vi "Buncher.vi"() -> ()   [LabVIEW 2014, in "Panels.lvlib"]
uses:
  Panels.lvlib
  CSlibraries-extern/DimLVEvent/DimIndicators/DimIndicators.lvlib
  CSlibraries/UtilityLib/UtilityLib.lvlib
  CS_Core/CSSystem/CoreLib/CoreLib.lvlib
  CSlibraries/UtilityLib/UtilityLib.valueStatus.ctl
  CS_Core/CSSystem/CoreLib/CoreLib.string 2 byte array.vi
  CSlibraries-extern/DimLVEvent/LVDimInterface/LVDimInterface.lvlib
  Instance           1 15Saved   Buncher .vi
  CS_Core/CSSystem/CoreLib/CoreLib.double 2 byte array.vi
  CS_Core/CSSystem/CoreLib/CoreLib.short 2 byte array.vi
  CSlibraries-extern/DimLVEvent/DimIndicators/DimIndicators.numericType.ctl
  CS_Core/BaseProcess/BaseProcess.descriptor string definition.ctl
  CS_Core/BaseProcess/BaseProcess.lvlib
  CS_Core/CSSystem/CoreDefs/CoreDefs.rawDataType.ctl
  CS_Core/CSSystem/CoreDefs/CoreDefs.call_type.ctl
  CSlibraries-extern/DimLVEvent/DimIndicators/DimIndicators.numericArrayType.ctl
  CSlibraries-extern/DimLVEvent/DimIndicators/DimIndicators.anyType.ctl
panel:
  in  "ListOfBases_Data":T1={"data"="NOLINK", "no link"=TRUE, "quality"=-1, "timeStamp"=0.0}
  in  "AmpCool":bool
  in  "AmpMicro":bool
  in  "AmpBun":bool
  in  "PercentNeon_SetValueInfoData":T2={"data"=[], "no link"=TRUE, "quality"=-1, "timeStamp"=0.0}
  in  "PercentNeon_SetData":T2={"data"=[], "no link"=TRUE, "quality"=-1, "timeStamp"=0.0}
  in  "PercentNeon":dbl=inf
  in  "SetFileLocation_Data":T1={"data"="NOLINK", "no link"=TRUE, "quality"=-1, "timeStamp"=0.0}
  in  "CoolPress":bool
  out "CoolPress_Mon":dbl=inf format="%.4f"
  in  "bunBase_SetValueInfoData":T2={"data"=[], "no link"=TRUE, "quality"=-1, "timeStamp"=0.0}
  in  "BunDefY_SetValueInfoData":T2={"data"=[], "no link"=TRUE, "quality"=-1, "timeStamp"=0.0}
  in  "BunDefX_SetValueInfoData":T2={"data"=[], "no link"=TRUE, "quality"=-1, "timeStamp"=0.0}
  in  "DCCool":bool
  in  "DCBun":bool
  in  "DCMicro":bool
  in  "ExBun1Eject":bool
  in  "ExBun1Cool":bool
  in  "Trap7Eject":bool
  in  "Trap7Cool":bool
  in  "Trap6Eject":bool
  in  "Trap6Cool":bool
  in  "Trap5Eject":bool
  in  "Trap5Cool":bool
  in  "Trap4Eject":bool
  in  "Trap4Cool":bool
  in  "Trap3Eject":bool
  in  "Trap3Cool":bool
  in  "Trap2Eject":bool
  in  "Trap2Cool":bool
  in  "Trap1Eject":bool
  in  "Trap1Cool":bool
  in  "BunDefY":bool
  in  "BunLens":bool
  in  "TranTube":bool
  in  "BunDefX":bool
  in  "DefLens":bool
  in  "ExBun2":bool
  in  "StartBun":bool
  in  "EndCool":bool
  in  "InjTunnel":bool
  in  "MicWedge2":bool
  in  "MicWedge1":bool
  in  "CoolWedge2":bool
  in  "CoolWedge1":bool
  in  "RetDisk2":bool
  in  "RetDisk1":bool
  in  "CoolPress_SetValueInfoData":T2={"data"=[], "no link"=TRUE, "quality"=-1, "timeStamp"=0.0}
  in  "CoolPress_SetData":T2={"data"=[], "no link"=TRUE, "quality"=-1, "timeStamp"=0.0}
  in  "CoolPress_MonData":T3={"data"=inf, "no link"=TRUE, "quality"=-1, "timeStamp"=0.0}
  in  "BunDefY_SetData":T2={"data"=[0.0, 0.0, 0.0, 0.0], "no link"=FALSE, "quality"=0, "timeStamp"=3268148655.414}
  in  "ExBun1Cool_SetValueInfoData":T2={"data"=[-399.9, 398.5, 0.0], "no link"=FALSE, "quality"=0, "timeStamp"=3268148655.43}
  in  "ExBun1Eject_SetValueInfoData":T2={"data"=[-401.1, 400.3, 0.0], "no link"=FALSE, "quality"=0, "timeStamp"=3268148655.43}
  in  "ExBun1Cool_SetData":T2={"data"=[0.0, 0.0, 0.0, 0.0], "no link"=FALSE, "quality"=0, "timeStamp"=3268148655.43}
  in  "ExBun1Eject_SetData":T2={"data"=[0.0, 0.0, 0.0, 0.0], "no link"=FALSE, "quality"=0, "timeStamp"=3268148655.414}
  in  "ExBun1Cool_MonData":T3={"data"=inf, "no link"=FALSE, "quality"=1, "timeStamp"=3268148655.399}
  in  "ExBun1Eject_MonData":T3={"data"=inf, "no link"=FALSE, "quality"=1, "timeStamp"=3268148655.399}
  in  "Trap7Eject_SetValueInfoData":T2={"data"=[-400.0, 400.0, 0.0], "no link"=FALSE, "quality"=0, "timeStamp"=3268148655.446}
  in  "Trap6Eject_SetValueInfoData":T2={"data"=[-400.0, 400.0, 0.0], "no link"=FALSE, "quality"=0, "timeStamp"=3268148655.446}
  in  "Trap5Eject_SetValueInfoData":T2={"data"=[-120.4, 119.2, 0.0], "no link"=FALSE, "quality"=0, "timeStamp"=3268148655.446}
  in  "Trap4Eject_SetValueInfoData":T2={"data"=[-400.0, 400.0, 0.0], "no link"=FALSE, "quality"=0, "timeStamp"=3268148655.446}
  in  "Trap3Eject_SetValueInfoData":T2={"data"=[-121.1, 120.3, 0.0], "no link"=FALSE, "quality"=0, "timeStamp"=3268148655.446}
  in  "Trap2Eject_SetValueInfoData":T2={"data"=[-120.0, 118.7, 0.0], "no link"=FALSE, "quality"=0, "timeStamp"=3268148655.446}
  in  "Trap1Eject_SetValueInfoData":T2={"data"=[-120.7, 119.5, 0.0], "no link"=FALSE, "quality"=0, "timeStamp"=3268148655.43}
  in  "Trap4Cool_SetValueInfoData":T2={"data"=[-400.0, 400.0, 0.0], "no link"=FALSE, "quality"=0, "timeStamp"=3268148655.43}
  in  "Trap3Cool_SetValueInfoData":T2={"data"=[-120.9, 119.8, 0.0], "no link"=FALSE, "quality"=0, "timeStamp"=3268148655.43}
  in  "Trap2Cool_SetValueInfoData":T2={"data"=[-119.2, 118.2, 0.0], "no link"=FALSE, "quality"=0, "timeStamp"=3268148655.43}
  in  "Trap1Cool_SetValueInfoData":T2={"data"=[-120.5, 119.3, 0.0], "no link"=FALSE, "quality"=0, "timeStamp"=3268148655.43}
  in  "Trap7Cool_SetValueInfoData":T2={"data"=[-400.0, 400.0, 0.0], "no link"=FALSE, "quality"=0, "timeStamp"=3268148655.43}
  in  "Trap6Cool_SetValueInfoData":T2={"data"=[-400.0, 400.0, 0.0], "no link"=FALSE, "quality"=0, "timeStamp"=3268148655.43}
  in  "Trap5Cool_SetValueInfoData":T2={"data"=[-120.4, 119.5, 0.0], "no link"=FALSE, "quality"=0, "timeStamp"=3268148655.43}
  in  "Trap7Eject_SetData":T2={"data"=[0.0, 0.0, 0.0, 0.0], "no link"=FALSE, "quality"=0, "timeStamp"=3268148655.414}
  in  "Trap6Eject_SetData":T2={"data"=[0.0, 0.0, 0.0, 0.0], "no link"=FALSE, "quality"=0, "timeStamp"=3268148655.414}
  in  "Trap5Eject_SetData":T2={"data"=[], "no link"=TRUE, "quality"=-1, "timeStamp"=0.0}
  in  "Trap4Eject_SetData":T2={"data"=[0.0, 0.0, 0.0, 0.0], "no link"=FALSE, "quality"=0, "timeStamp"=3268148655.414}
  in  "Trap1Eject_SetData":T2={"data"=[0.0, 0.0, 0.0, 0.0], "no link"=FALSE, "quality"=0, "timeStamp"=3268148655.414}
  in  "Trap2Eject_SetData":T2={"data"=[0.0, 0.0, 0.0, 0.0], "no link"=FALSE, "quality"=0, "timeStamp"=3268148655.414}
  in  "Trap6Cool_SetData":T2={"data"=[0.0, 0.0, 0.0, 0.0], "no link"=FALSE, "quality"=0, "timeStamp"=3268148655.414}
  in  "Trap7Cool_SetData":T2={"data"=[0.0, 0.0, 0.0, 0.0], "no link"=FALSE, "quality"=0, "timeStamp"=3268148655.414}
  in  "Trap4Cool_SetData":T2={"data"=[0.0, 0.0, 0.0, 0.0], "no link"=FALSE, "quality"=0, "timeStamp"=3268148655.414}
  in  "Trap5Cool_SetData":T2={"data"=[0.0, 0.0, 0.0, 0.0], "no link"=FALSE, "quality"=0, "timeStamp"=3268148655.414}
  in  "Trap3Eject_SetData":T2={"data"=[0.0, 0.0, 0.0, 0.0], "no link"=FALSE, "quality"=0, "timeStamp"=3268148655.414}
  in  "Trap3Cool_SetData":T2={"data"=[0.0, 0.0, 0.0, 0.0], "no link"=FALSE, "quality"=0, "timeStamp"=3268148655.414}
  in  "Trap1Cool_SetData":T2={"data"=[0.0, 0.0, 0.0, 0.0], "no link"=FALSE, "quality"=0, "timeStamp"=3268148655.414}
  in  "Trap2Cool_SetData":T2={"data"=[0.0, 0.0, 0.0, 0.0], "no link"=FALSE, "quality"=0, "timeStamp"=3268148655.414}
  in  "Trap7Eject_MonData":T3={"data"=inf, "no link"=FALSE, "quality"=1, "timeStamp"=3268148655.399}
  in  "Trap5Eject_MonData":T3={"data"=inf, "no link"=FALSE, "quality"=1, "timeStamp"=3268148655.399}
  in  "Trap6Eject_MonData":T3={"data"=inf, "no link"=FALSE, "quality"=1, "timeStamp"=3268148655.399}
  in  "Trap3Eject_MonData":T3={"data"=inf, "no link"=FALSE, "quality"=1, "timeStamp"=3268148655.399}
  in  "Trap4Eject_MonData":T3={"data"=inf, "no link"=FALSE, "quality"=1, "timeStamp"=3268148655.399}
  in  "Trap1Eject_MonData":T3={"data"=inf, "no link"=FALSE, "quality"=1, "timeStamp"=3268148655.399}
  in  "Trap2Eject_MonData":T3={"data"=inf, "no link"=FALSE, "quality"=1, "timeStamp"=3268148655.399}
  in  "Trap6Cool_MonData":T3={"data"=inf, "no link"=FALSE, "quality"=1, "timeStamp"=3268148655.399}
  in  "Trap7Cool_MonData":T3={"data"=inf, "no link"=FALSE, "quality"=1, "timeStamp"=3268148655.399}
  in  "Trap1Cool_MonData":T3={"data"=inf, "no link"=FALSE, "quality"=1, "timeStamp"=3268148655.399}
  in  "Trap3Cool_MonData":T3={"data"=inf, "no link"=FALSE, "quality"=1, "timeStamp"=3268148655.399}
  in  "Trap2Cool_MonData":T3={"data"=inf, "no link"=FALSE, "quality"=1, "timeStamp"=3268148655.399}
  in  "BunDefX_MonData":T3={"data"=0.0, "no link"=FALSE, "quality"=0, "timeStamp"=3268148655.399}
  in  "Trap4Cool_MonData":T3={"data"=inf, "no link"=FALSE, "quality"=1, "timeStamp"=3268148655.399}
  in  "Trap5Cool_MonData":T3={"data"=inf, "no link"=FALSE, "quality"=1, "timeStamp"=3268148655.399}
  in  "Thermocouple3_MonData":T3={"data"=inf, "no link"=FALSE, "quality"=1, "timeStamp"=3268148655.399}
  in  "Thermocouple4_MonData":T3={"data"=inf, "no link"=FALSE, "quality"=1, "timeStamp"=3268148655.399}
  in  "BunDefY_MonData":T3={"data"=0.0, "no link"=FALSE, "quality"=0, "timeStamp"=3268148655.399}
  in  "InjTunnel_MonData":T3={"data"=inf, "no link"=FALSE, "quality"=1, "timeStamp"=3268148655.383}
  in  "CoolWedge1_MonData":T3={"data"=inf, "no link"=FALSE, "quality"=1, "timeStamp"=3268148655.383}
  in  "CoolWedge2_MonData":T3={"data"=inf, "no link"=FALSE, "quality"=1, "timeStamp"=3268148655.383}
  in  "EndCool_MonData":T3={"data"=inf, "no link"=FALSE, "quality"=1, "timeStamp"=3268148655.383}
  in  "DCCool_MonData":T3={"data"=inf, "no link"=FALSE, "quality"=1, "timeStamp"=3268148655.383}
  in  "AmpCool_MonData":T3={"data"=inf, "no link"=FALSE, "quality"=1, "timeStamp"=3268148655.383}
  in  "FreqCool_MonData":T3={"data"=inf, "no link"=FALSE, "quality"=1, "timeStamp"=3268148655.383}
  in  "MicWedge1_MonData":T3={"data"=inf, "no link"=FALSE, "quality"=1, "timeStamp"=3268148655.383}
  in  "MicWedge2_MonData":T3={"data"=inf, "no link"=FALSE, "quality"=1, "timeStamp"=3268148655.383}
  in  "StartBun_MonData":T3={"data"=inf, "no link"=FALSE, "quality"=1, "timeStamp"=3268148655.383}
  in  "DCMicro_MonData":T3={"data"=inf, "no link"=FALSE, "quality"=1, "timeStamp"=3268148655.383}
  in  "RetDisk2_MonData":T3={"data"=inf, "no link"=FALSE, "quality"=1, "timeStamp"=3268148655.383}
  in  "RetDisk1_MonData":T3={"data"=inf, "no link"=FALSE, "quality"=1, "timeStamp"=3268148655.383}
  in  "Thermocouple2_MonData":T3={"data"=inf, "no link"=FALSE, "quality"=1, "timeStamp"=3268148655.383}
  in  "Thermocouple1_MonData":T3={"data"=inf, "no link"=FALSE, "quality"=1, "timeStamp"=3268148655.383}
  in  "bunBase_MonData":T3={"data"=inf, "no link"=TRUE, "quality"=-1, "timeStamp"=0.0}
  in  "ExBun2_MonData":T3={"data"=inf, "no link"=FALSE, "quality"=1, "timeStamp"=3268148655.383}
  in  "TranTube_MonData":T3={"data"=inf, "no link"=FALSE, "quality"=1, "timeStamp"=3268148655.383}
  in  "AmpBun_MonData":T3={"data"=inf, "no link"=FALSE, "quality"=1, "timeStamp"=3268148655.383}
  in  "DCBun_MonData":T3={"data"=inf, "no link"=FALSE, "quality"=1, "timeStamp"=3268148655.383}
  in  "PhaseMicro_MonData":T3={"data"=inf, "no link"=FALSE, "quality"=1, "timeStamp"=3268148655.383}
  in  "AmpMicro_MonData":T3={"data"=inf, "no link"=FALSE, "quality"=1, "timeStamp"=3268148655.383}
  in  "PhaseBun_MonData":T3={"data"=inf, "no link"=FALSE, "quality"=1, "timeStamp"=3268148655.383}
  in  "DefLens_MonData":T3={"data"=inf, "no link"=FALSE, "quality"=1, "timeStamp"=3268148655.383}
  in  "BunLens_MonData":T3={"data"=inf, "no link"=FALSE, "quality"=1, "timeStamp"=3268148655.399}
  out "ExBun1Eject_Mon":dbl=inf format="%.4f"
  out "ExBun1Cool_Mon":dbl=inf format="%.4f"
  out "Trap7Eject_Mon":dbl=inf format="%.4f"
  out "Trap7Cool_Mon":dbl=inf format="%.4f"
  out "Trap6Eject_Mon":dbl=inf format="%.4f"
  out "Trap6Cool_Mon":dbl=inf format="%.4f"
  out "Trap5Eject_Mon":dbl=inf format="%.4f"
  out "Trap5Cool_Mon":dbl=inf format="%.4f"
  out "Trap4Eject_Mon":dbl=inf format="%.4f"
  out "Trap4Cool_Mon":dbl=inf format="%.4f"
  out "Trap3Eject_Mon":dbl=inf format="%.4f"
  out "Trap3Cool_Mon":dbl=inf format="%.4f"
  out "Trap2Eject_Mon":dbl=inf format="%.4f"
  out "Trap2Cool_Mon":dbl=inf format="%.4f"
  out "Trap1Eject_Mon":dbl=inf format="%.4f"
  out "Trap1Cool_Mon":dbl=inf format="%.4f"
  out "BunDefX_Mon":dbl format="%.4f"
  out "BunDefY_Mon":dbl format="%.4f"
  in  "bunBase_SetValueInfoData":T2={"data"=[], "no link"=TRUE, "quality"=-1, "timeStamp"=0.0}
  in  "RetDisk1_SetValueInfoData":T2={"data"=[0.3, 1481.2, 0.0], "no link"=FALSE, "quality"=0, "timeStamp"=3268148655.43}
  in  "bunBase_SetData":T2={"data"=[], "no link"=TRUE, "quality"=-1, "timeStamp"=0.0}
  in  "RetDisk1_SetData":T2={"data"=[1.0, 0.0, 0.0, 0.0], "no link"=FALSE, "quality"=0, "timeStamp"=3268148655.399}
  out "Thermocouple4_Mon":dbl=inf format="%.4f"
  out "Thermocouple3_Mon":dbl=inf format="%.4f"
  out "PhaseBun_Mon":dbl=inf format="%.4f"
  in  "RetDisk2_SetData":T2={"data"=[0.0, 0.0, 0.0, 0.0], "no link"=FALSE, "quality"=0, "timeStamp"=3268148655.399}
  in  "BunLens_SetValueInfoData":T2={"data"=[1.2, 4695.6, -1.0], "no link"=FALSE, "quality"=0, "timeStamp"=3268148655.43}
  in  "DefLens_SetValueInfoData":T2={"data"=[0.0, 2075.4, -1.0], "no link"=FALSE, "quality"=0, "timeStamp"=3268148655.43}
  in  "TranTube_SetValueInfoData":T2={"data"=[], "no link"=TRUE, "quality"=-1, "timeStamp"=0.0}
  in  "ExBun2_SetValueInfoData":T2={"data"=[0.0, 750.0, 0.0], "no link"=FALSE, "quality"=0, "timeStamp"=3268148655.43}
  in  "PhaseBun_SetValueInfoData":T2={"data"=[0.0, 10.0, -1.0], "no link"=FALSE, "quality"=0, "timeStamp"=3268148655.43}
  in  "AmpBun_SetValueInfoData":T2={"data"=[0.0, 200.0, -1.0], "no link"=FALSE, "quality"=0, "timeStamp"=3268148655.43}
  in  "DCBun_SetValueInfoData":T2={"data"=[], "no link"=TRUE, "quality"=-1, "timeStamp"=0.0}
  in  "PhaseMicro_SetValueInfoData":T2={"data"=[0.0, 10.0, -1.0], "no link"=FALSE, "quality"=0, "timeStamp"=3268148655.43}
  in  "AmpMicro_SetValueInfoData":T2={"data"=[0.0, 10.0, -1.0], "no link"=FALSE, "quality"=0, "timeStamp"=3268148655.43}
  in  "DCMicro_SetValueInfoData":T2={"data"=[-119.7, 119.1, 0.0], "no link"=FALSE, "quality"=0, "timeStamp"=3268148655.43}
  in  "BunLens_SetData":T2={"data"=[0.0, 0.0, 0.0, 0.0], "no link"=FALSE, "quality"=1, "timeStamp"=3268148655.414}
  in  "DefLens_SetData":T2={"data"=[0.0, 0.0, 0.0, 0.0], "no link"=FALSE, "quality"=0, "timeStamp"=3268148655.414}
  in  "TranTube_SetData":T2={"data"=[], "no link"=TRUE, "quality"=-1, "timeStamp"=0.0}
  in  "ExBun2_SetData":T2={"data"=[0.0, 0.0, 0.0, 0.0], "no link"=FALSE, "quality"=0, "timeStamp"=3268148655.414}
  in  "PhaseBun_SetData":T2={"data"=[0.0, 0.0, 0.0, 0.0], "no link"=FALSE, "quality"=0, "timeStamp"=3268148655.414}
  in  "AmpBun_SetData":T2={"data"=[0.0, 0.0, 0.0, 0.0], "no link"=FALSE, "quality"=0, "timeStamp"=3268148655.414}
  in  "DCBun_SetData":T2={"data"=[0.0, 0.0, 0.0, 0.0], "no link"=FALSE, "quality"=0, "timeStamp"=3268148655.414}
  in  "PhaseMicro_SetData":T2={"data"=[0.0, 0.0, 0.0, 0.0], "no link"=FALSE, "quality"=0, "timeStamp"=3268148655.414}
  in  "AmpMicro_SetData":T2={"data"=[0.0, 0.0, 0.0, 0.0], "no link"=FALSE, "quality"=0, "timeStamp"=3268148655.414}
  out "AmpMicro_Mon":dbl=inf format="%.4f"
  out "ExBun2_Mon":dbl=inf format="%.4f"
  out "StartBun_Mon":dbl=inf format="%.4f"
  out "DefLens_Mon":dbl=inf format="%.4f"
  out "DCBun_Mon":dbl=inf format="%.4f"
  out "MicWedge1_Mon":dbl=inf format="%.4f"
  out "BunLens_Mon":dbl=inf format="%.4f"
  out "EndCool_Mon":dbl=inf format="%.4f"
  out "TranTube_Mon":dbl=inf format="%.4f"
  out "AmpCool_Mon":dbl=inf format="%.4f"
  out "Thermocouple1_Mon":dbl=inf format="%.4f"
  out "Thermocouple2_Mon":dbl=inf format="%.4f"
  in  "StartBun_SetValueInfoData":T2={"data"=[-120.2, 119.2, 0.0], "no link"=FALSE, "quality"=0, "timeStamp"=3268148655.43}
  in  "DCMicro_SetData":T2={"data"=[0.0, 0.0, 0.0, 0.0], "no link"=FALSE, "quality"=0, "timeStamp"=3268148655.414}
  in  "MicWedge2_SetValueInfoData":T2={"data"=[-121.2, 119.6, 0.0], "no link"=FALSE, "quality"=0, "timeStamp"=3268148655.43}
  in  "StartBun_SetData":T2={"data"=[0.0, 0.0, 0.0, 0.0], "no link"=FALSE, "quality"=0, "timeStamp"=3268148655.414}
  out "FreqCool_Mon":dbl=inf format="%.4f"
  out "InjTunnel_Mon":dbl=inf format="%.4f"
  out "i ref out":refnum<vi>
  in  "Last Loaded File_Data":T1
  out "FileUpToDate":bool caption="Parameter Changed"
  in  "Close All Panels":bool
  in  "InjTunnel_SetValueInfoData":T2={"data"=[-117.0, 118.6, 0.0], "no link"=FALSE, "quality"=0, "timeStamp"=3268148655.43}
  in  "CoolWedge1_SetValueInfoData":T2={"data"=[-121.0, 119.3, 0.0], "no link"=FALSE, "quality"=0, "timeStamp"=3268148655.43}
  in  "CoolWedge2_SetValueInfoData":T2={"data"=[-120.6, 119.2, 0.0], "no link"=FALSE, "quality"=0, "timeStamp"=3268148655.43}
  in  "EndCool_SetValueInfoData":T2={"data"=[-120.1, 119.3, 0.0], "no link"=FALSE, "quality"=0, "timeStamp"=3268148655.43}
  in  "DCCool_SetValueInfoData":T2={"data"=[-117.9, 118.2, 0.0], "no link"=FALSE, "quality"=0, "timeStamp"=3268148655.43}
  in  "AmpCool_SetValueInfoData":T2={"data"=[0.0, 10.0, -1.0], "no link"=FALSE, "quality"=0, "timeStamp"=3268148655.43}
  in  "FreqCool_SetValueInfoData":T2={"data"=[0.0, 10.0, -1.0], "no link"=FALSE, "quality"=0, "timeStamp"=3268148655.43}
  in  "MicWedge1_SetValueInfoData":T2={"data"=[-121.3, 119.6, 0.0], "no link"=FALSE, "quality"=0, "timeStamp"=3268148655.43}
  in  "RetDisk2_SetValueInfoData":T2={"data"=[-398.3, 402.3, 0.0], "no link"=FALSE, "quality"=0, "timeStamp"=3268148655.43}
  in  "BunDefX_SetData":T2={"data"=[0.0, 0.0, 0.0, 0.0], "no link"=FALSE, "quality"=0, "timeStamp"=3268148655.414}
  in  "MicWedge1_SetData":T2={"data"=[], "no link"=TRUE, "quality"=-1, "timeStamp"=0.0}
  in  "FreqCool_SetData":T2={"data"=[0.0, 0.0, 0.0, 0.0], "no link"=FALSE, "quality"=0, "timeStamp"=3268148655.414}
  in  "AmpCool_SetData":T2={"data"=[0.0, 0.0, 0.0, 0.0], "no link"=FALSE, "quality"=0, "timeStamp"=3268148655.414}
  in  "DCCool_SetData":T2={"data"=[0.0, 0.0, 0.0, 0.0], "no link"=FALSE, "quality"=0, "timeStamp"=3268148655.414}
  in  "EndCool_SetData":T2={"data"=[0.0, 0.0, 0.0, 0.0], "no link"=FALSE, "quality"=0, "timeStamp"=3268148655.414}
  in  "CoolWedge2_SetData":T2={"data"=[0.0, 0.0, 0.0, 0.0], "no link"=FALSE, "quality"=0, "timeStamp"=3268148655.414}
  in  "CoolWedge1_SetData":T2={"data"=[0.0, 0.0, 0.0, 0.0], "no link"=FALSE, "quality"=0, "timeStamp"=3268148655.399}
  in  "InjTunnel_SetData":T2={"data"=[0.0, 0.0, 0.0, 0.0], "no link"=FALSE, "quality"=0, "timeStamp"=3268148655.399}
  in  "MicWedge2_SetData":T2={"data"=[], "no link"=TRUE, "quality"=-1, "timeStamp"=0.0}
  in  "call cluster in":T4={"Object"="", "Selector"="", "CallType"=enum."synchronous", "Async Object"="", "Async Selector"="", "Data Descriptor"="", "Data"=[], "Error #"=0, "Expire"=0}
  in  "bunBase":dbl=inf
  out "Last Loaded File":string
  in  "SetFileLocation":path=path "\\\\intranet\\Files/projects/lebit/Data Exchange/data/bunControl"
  out "CoolWedge1_Mon":dbl=inf format="%.4f"
  out "MicWedge2_Mon":dbl=inf format="%.4f"
  out "PhaseMicro_Mon":dbl=inf format="%.4f"
  out "RetDisk2_Mon":dbl=inf format="%.4f"
  out "AmpBun_Mon":dbl=inf format="%.4f"
  out "CoolWedge2_Mon":dbl=inf format="%.4f"
  out "DCCool_Mon":dbl=inf format="%.4f"
  out "DCMicro_Mon":dbl=inf format="%.4f"
  out "RetDisk1_Mon":dbl=inf format="%.4f"
  # "Parameter changed, data file is no longer up-to-date."
  # "Cool"
  # "Eject"
  # "Thermocouple3"
  # "Thermocouple1"
  # "Thermocouple4"
  # "Thermocouple2"
  # "Set CoolPress\nto zero before \nchanging \nPercentNeon"
  # "FreqCool"
  # "PhaseMicro"
  # "PhaseBun"
  # "Values in italic don't have a real monitor"
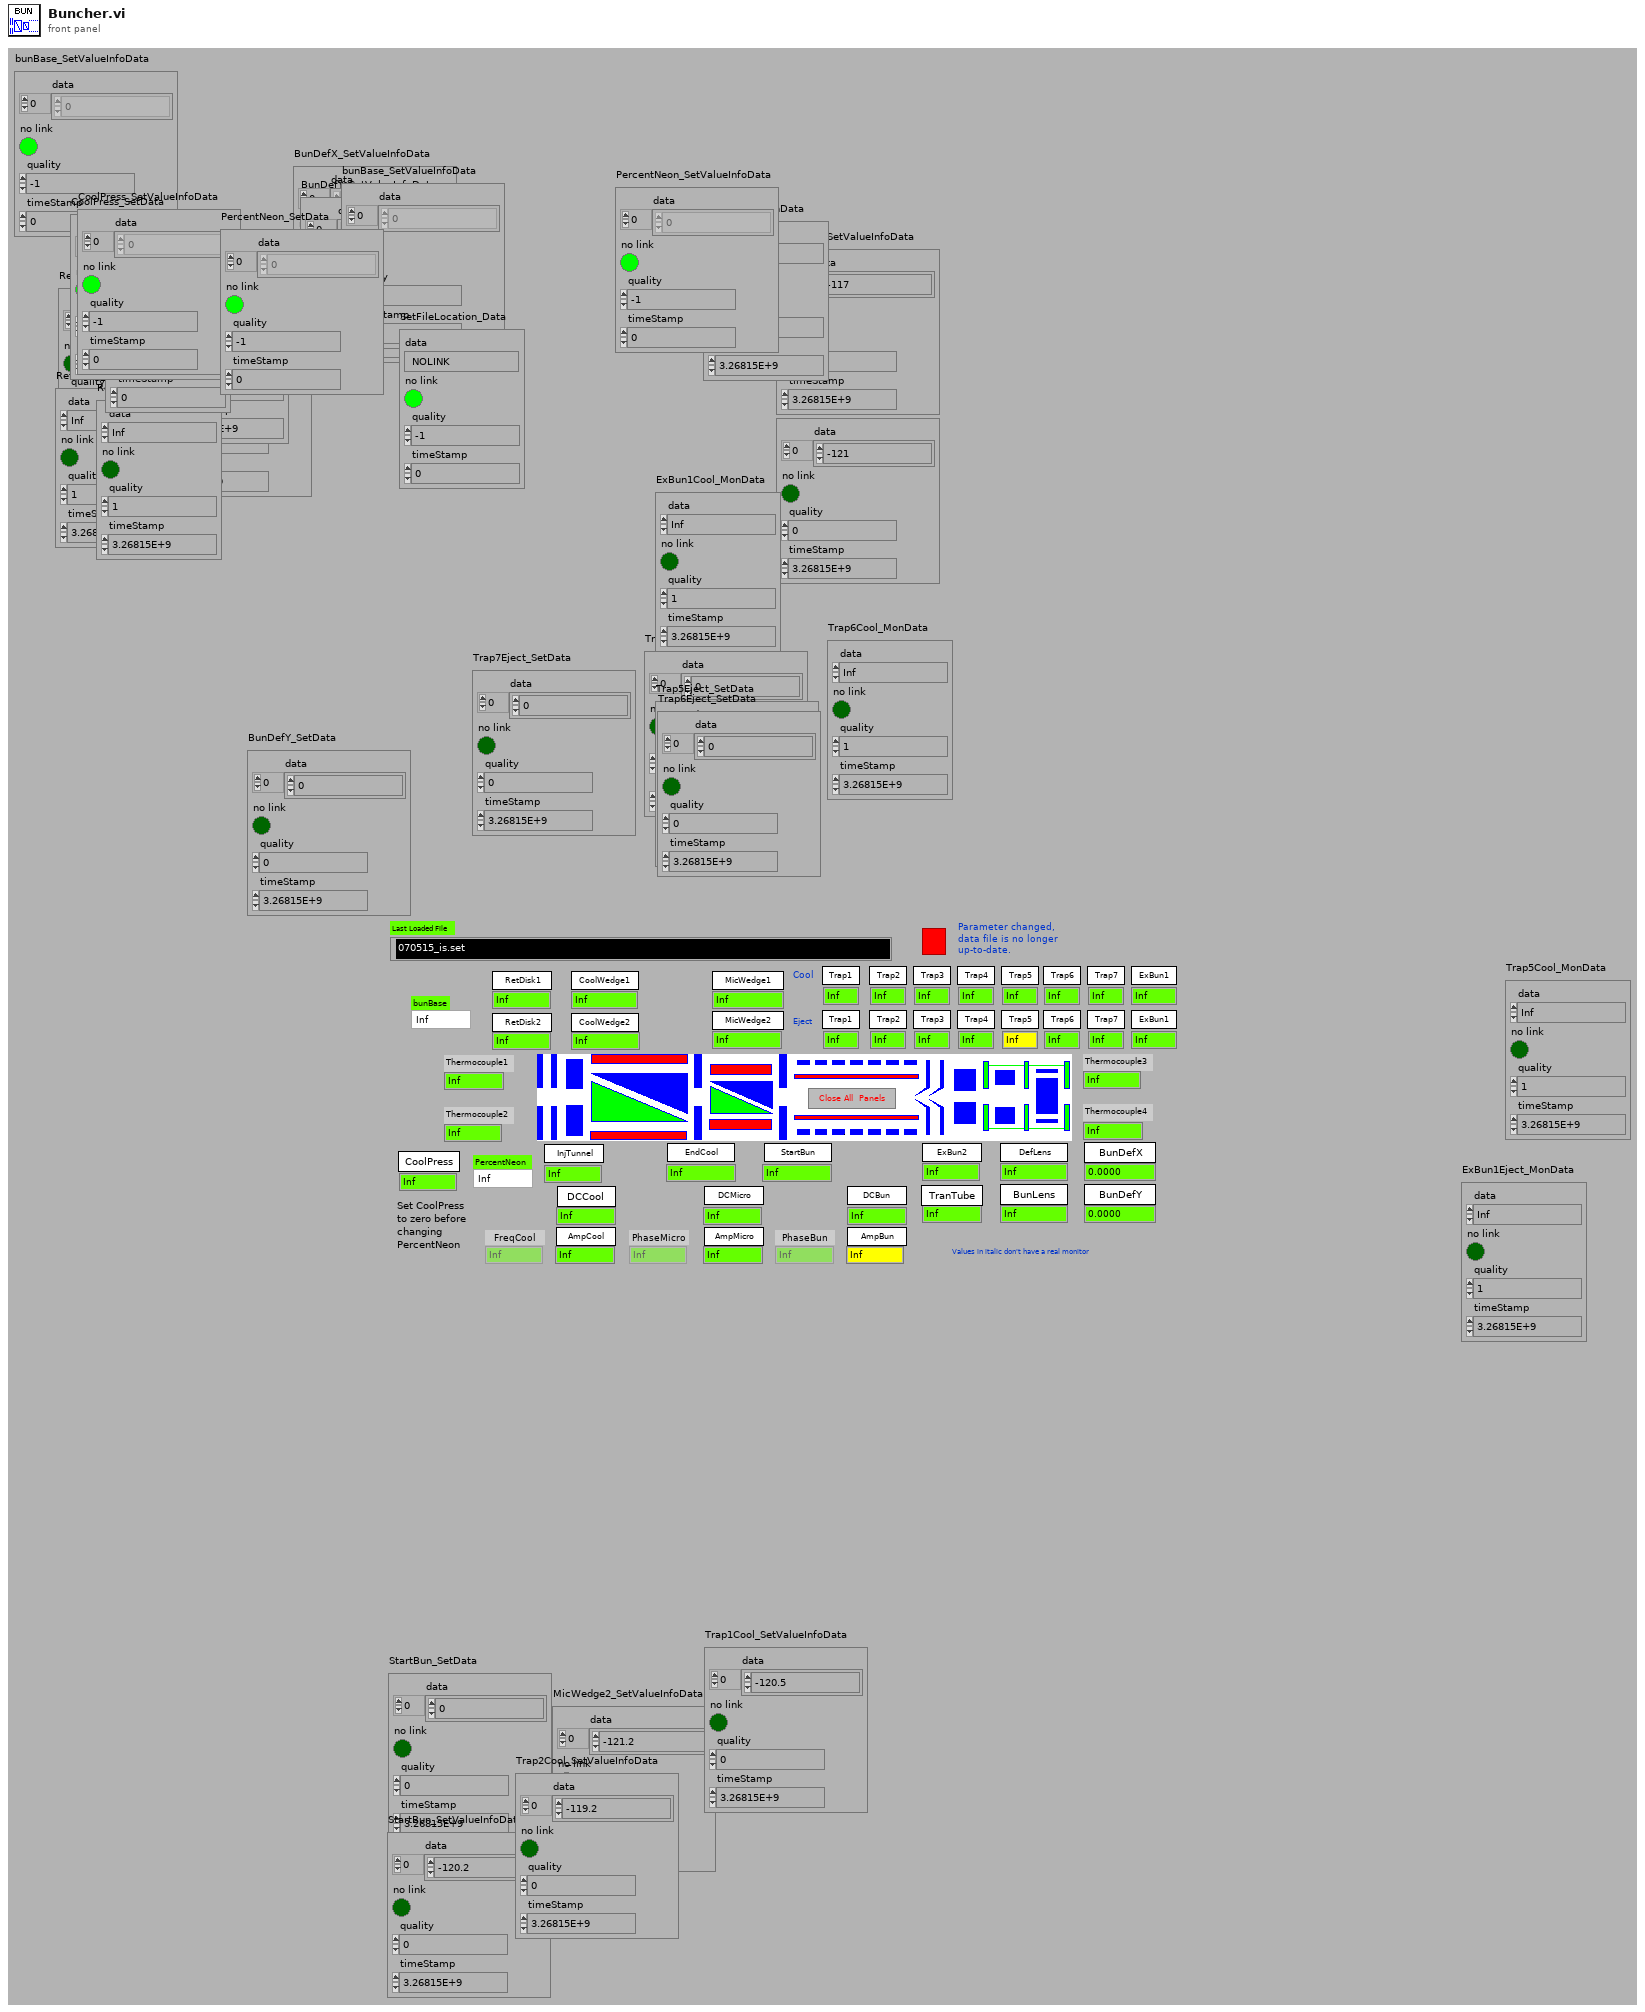
[diagram p1: front panel]
types:
  T1 = typedef "DimIndicators.lvlib/DimIndicators.anyType.ctl" = cluster{"data":string, "no link":bool, "quality":i32, "timeStamp":dbl}
  T2 = typedef "DimIndicators.lvlib/DimIndicators.numericArrayType.ctl" = cluster{"data":dbl[], "no link":bool, "quality":i32, "timeStamp":dbl}
  T3 = typedef "DimIndicators.lvlib/DimIndicators.numericType.ctl" = cluster{"data":dbl, "no link":bool, "quality":i32, "timeStamp":dbl}
  T4 = typedef "CoreDefs.call_type.ctl" = cluster{"Object":string, "Selector":string, "CallType":enum16{"simple", "synchronous", "asynchronous"}, "Async Object":string, "Async Selector":string, "Data Descriptor":T5, "Data":T6, "Error #":i32, "Expire":u32}
  T5 = typedef "BaseProcess.lvlib/BaseProcess.descriptor string definition.ctl" = string
  T6 = typedef "CoreDefs.rawDataType.ctl" = i8[]
  T7 = typedef "UtilityLib.lvlib/UtilityLib.valueStatus.ctl" = enum16{"no info available", "stand by/off", "on", "warning", "alarm/malfunction", "not implemented", "user action required", "important information", "system default", "control default", "indicator default", "button default"}
  T8 = cluster{"data":string, "no link":bool, "quality":i32, "timeStamp":dbl}
  T9 = cluster{"data":dbl[], "no link":bool, "quality":i32, "timeStamp":dbl}
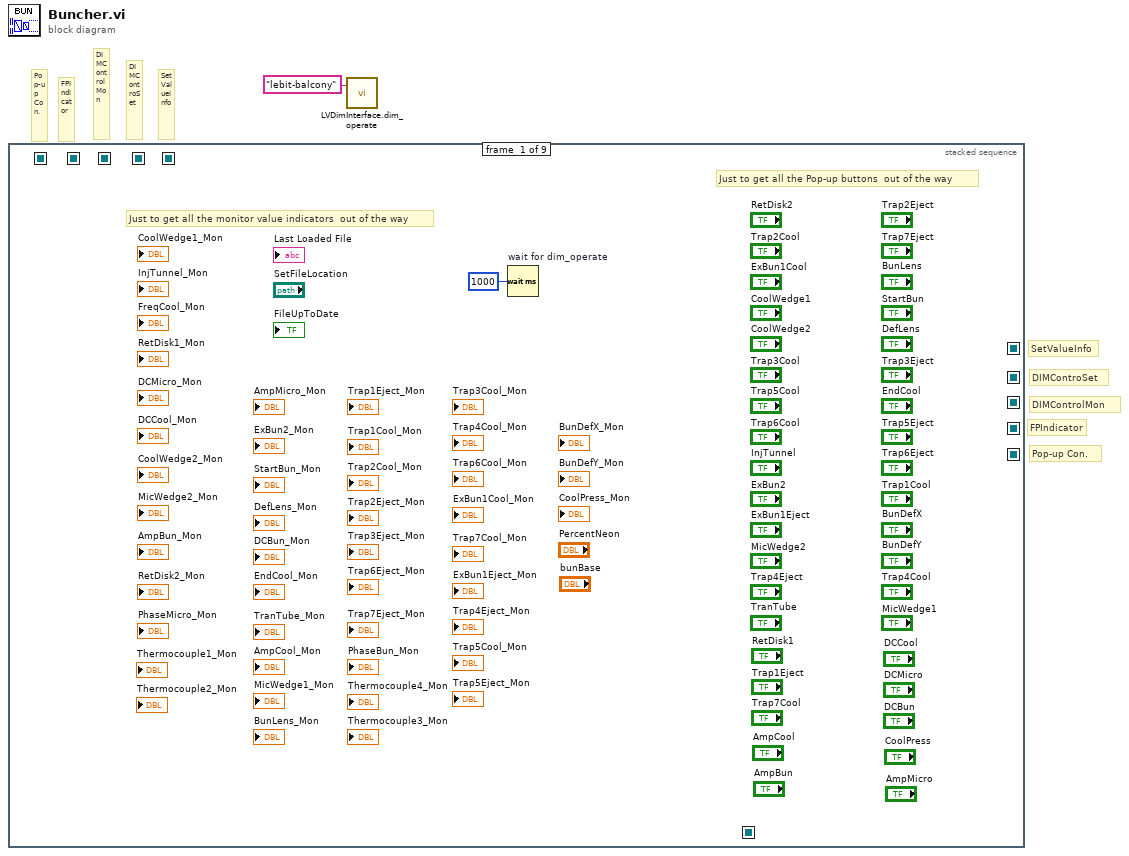
[diagram p0: block diagram]
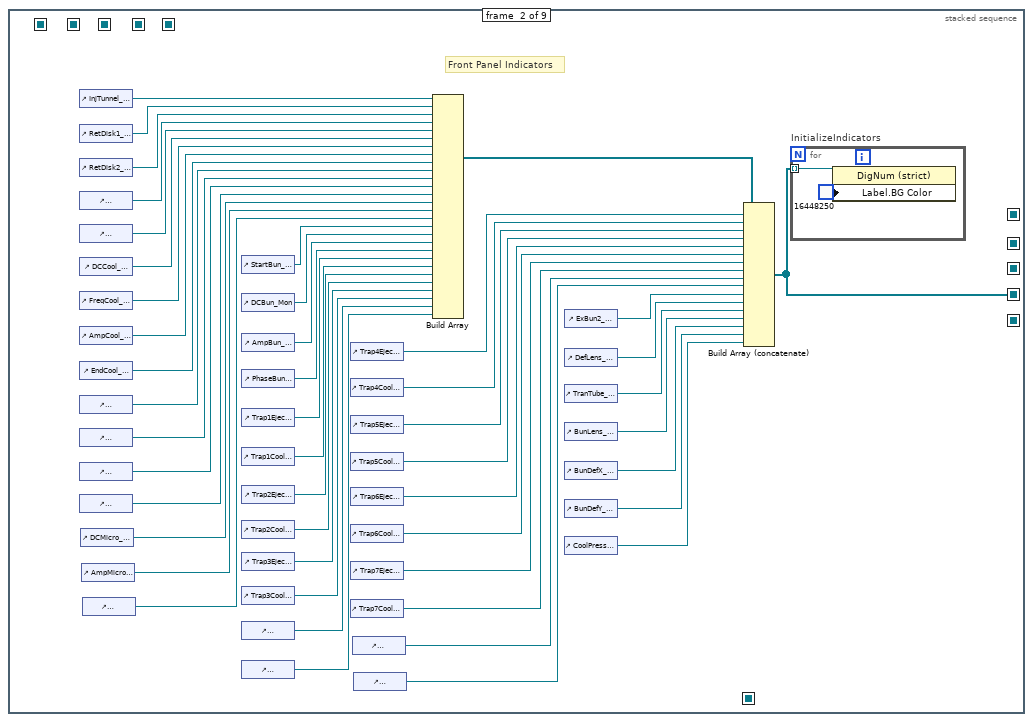
[diagram p2: hidden frame]
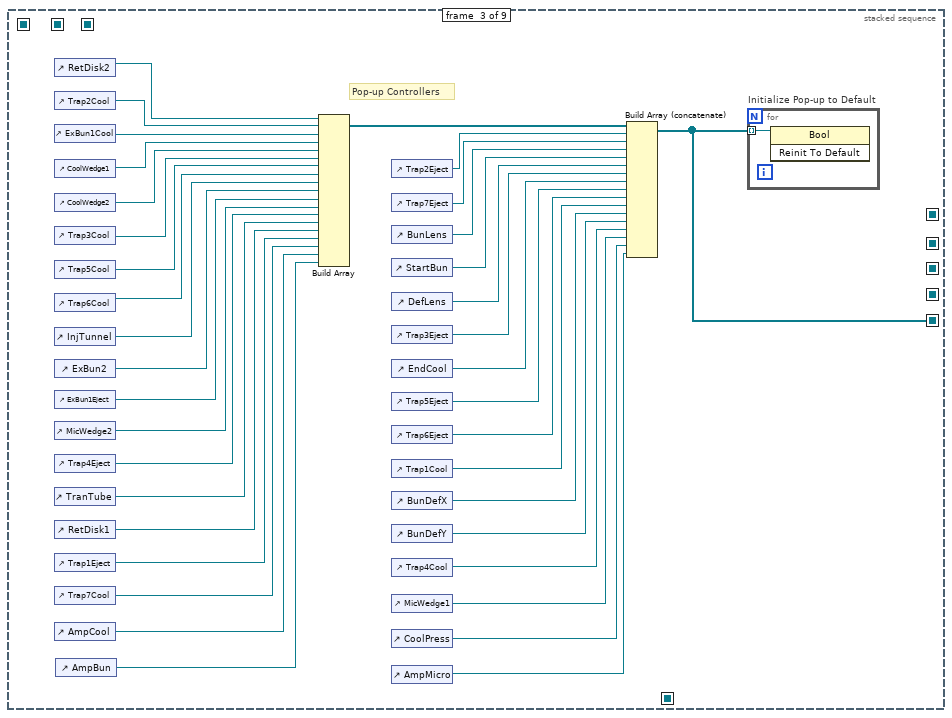
[diagram p3: hidden frame]
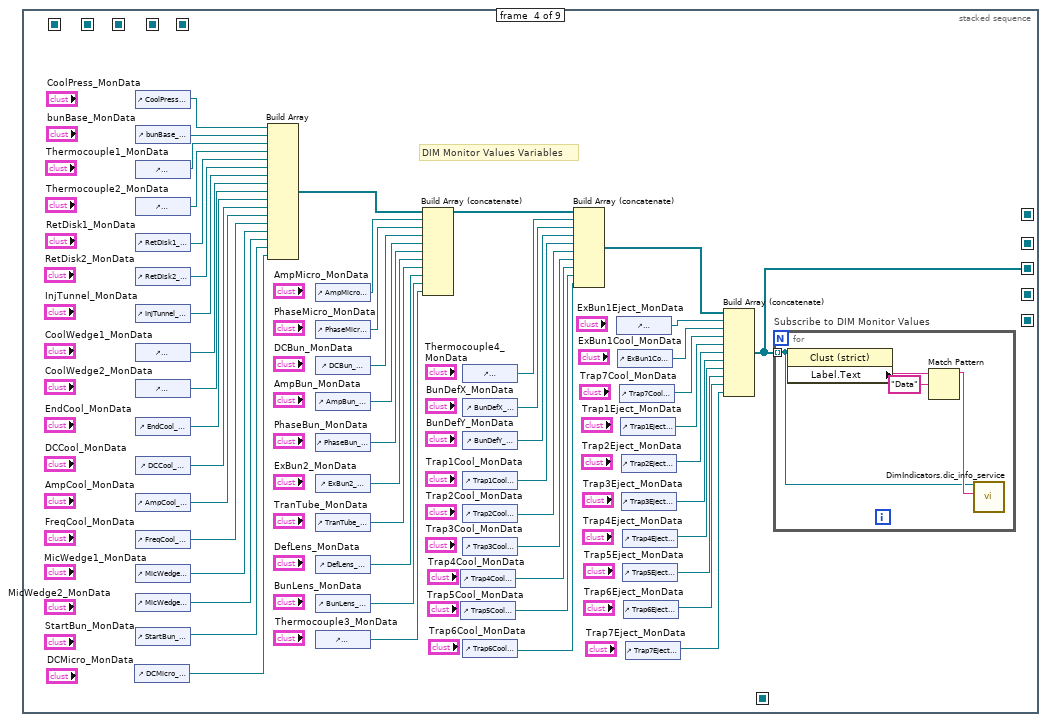
[diagram p4: hidden frame]
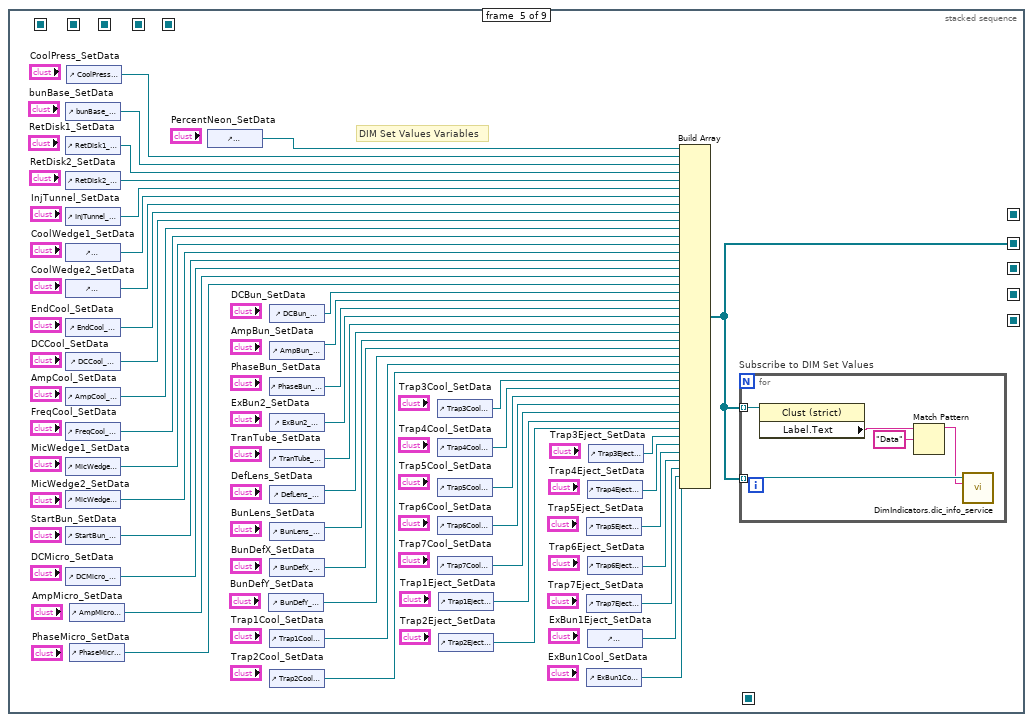
[diagram p5: hidden frame]
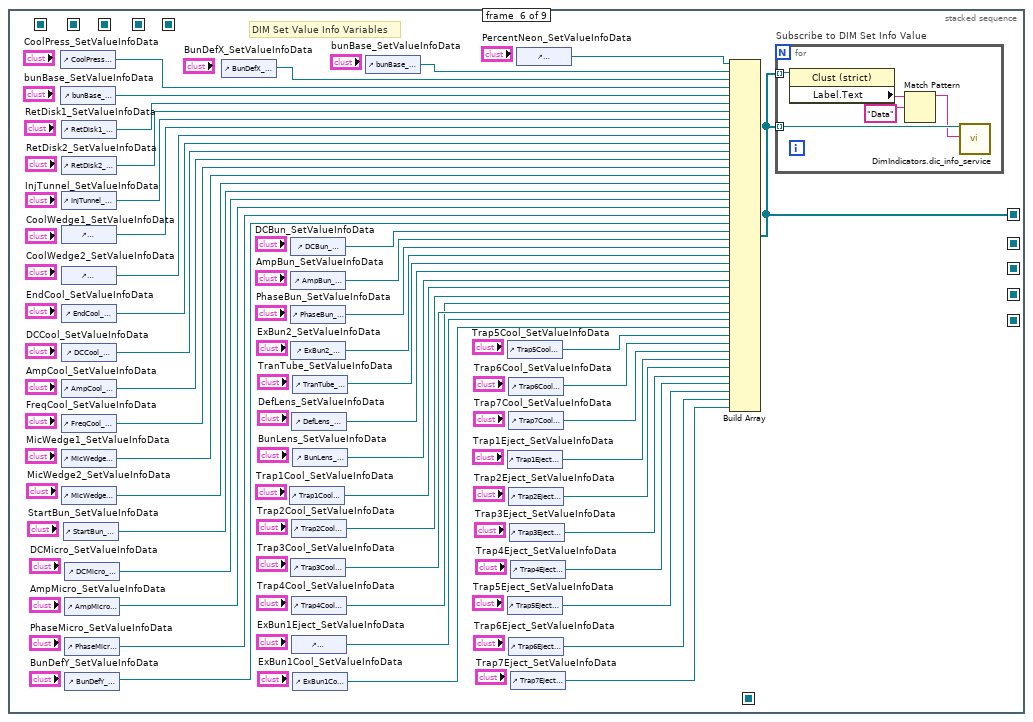
[diagram p6: hidden frame]
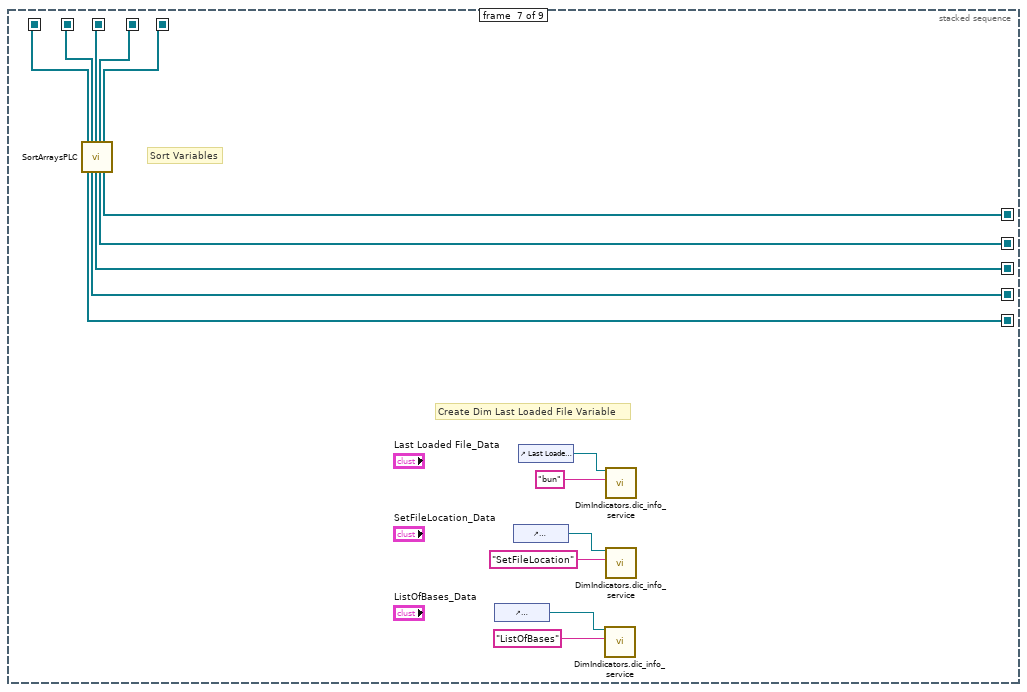
[diagram p7: hidden frame]
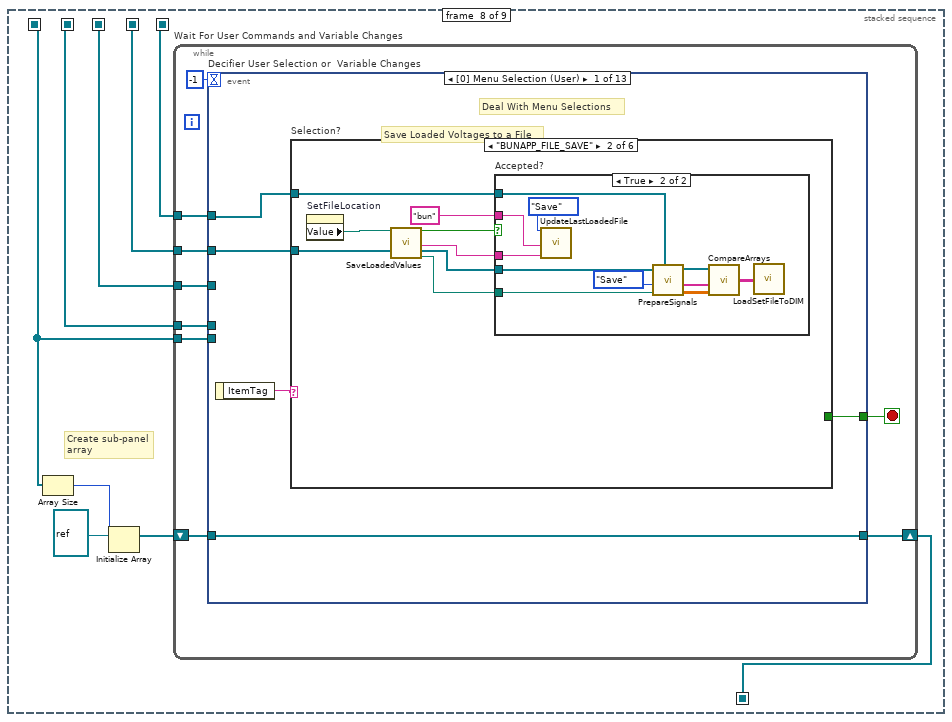
[diagram p8: hidden frame]
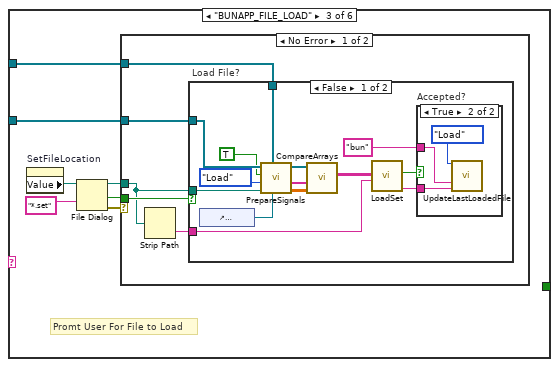
[diagram p11: hidden frame]
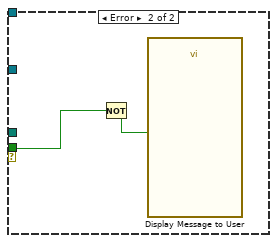
[diagram p14: hidden frame]
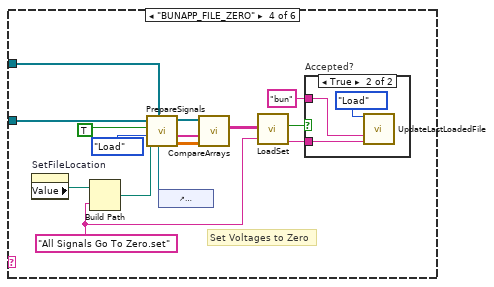
[diagram p15: hidden frame]
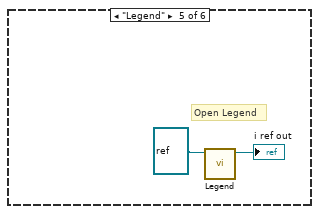
[diagram p17: hidden frame]
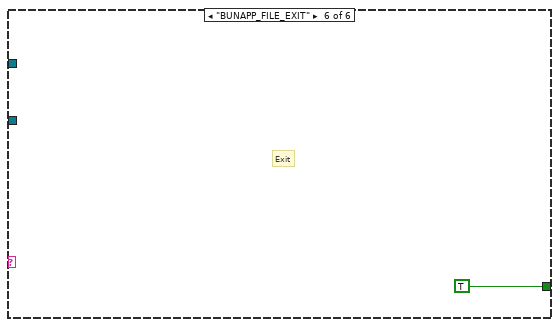
[diagram p18: hidden frame]
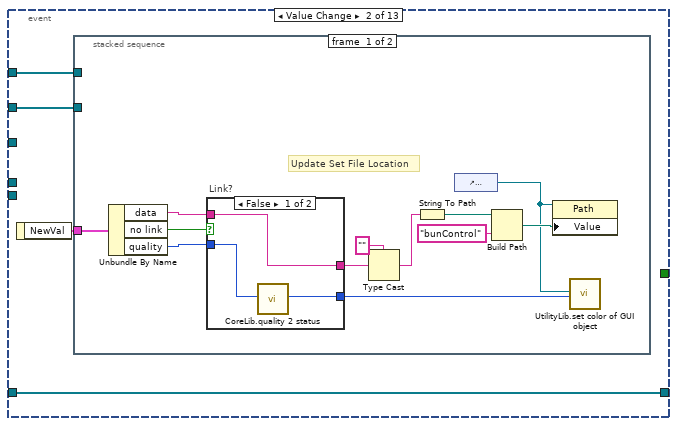
[diagram p19: hidden frame]
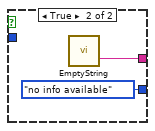
[diagram p20: hidden frame]
diagram:
  # "DIMControlMon"
  # "DIMControSet"
  # "SetValueInfo"
  # "Pop-up Con."
  # "FPIndicator"
  # "Pop-up Con."
  # "SetValueInfo"
  # "DIMControSet"
  # "DIMControlMon"
  # "FPIndicator"
  n1 = stacked-sequence {
    seq-local: [_ _ _ _ _ _ w250 _ _] -> [_ _ _ _ _ _ _ w264 _]
    seq-local: [_ _ _ _ _ _ w251 _ _] -> [_ _ _ _ _ _ _ w267 w562]
    seq-local: [_ _ _ _ _ _ _ w262 _] -> [_ _ _ _ _ _ _ _ w561]
    seq-local: [_ _ _ _ _ _ w252 _ _] -> [_ _ _ _ _ _ _ w261 w560]
    seq-local: [_ _ _ _ _ _ w253 _ _] -> [_ _ _ _ _ _ _ w260 w559]
    seq-local: [_ _ _ _ _ _ w249 _ _] -> [_ _ _ _ _ _ _ w259 _]
    seq-local: [_ w41 _ _ _ _ _ _ _] -> [_ _ _ _ _ _ w258 _ _]
    seq-local: [_ _ _ w90 _ _ _ _ _] -> [_ _ _ _ _ _ w256 _ _]
    seq-local: [_ _ _ _ _ w198 _ _ _] -> [_ _ _ _ _ _ w254 _ _]
    seq-local: [_ _ _ _ w145 _ _ _ _] -> [_ _ _ _ _ _ w255 _ _]
    seq-local: [_ _ w56 _ _ _ _ _ _] -> [_ _ _ _ _ _ w257 _ _]
    frame #0 {
      # "Just to get all the Pop-up buttons  out of the way"
      # "Just to get all the monitor value indicators  out of the way"
      n2 = Wait (ms) "wait for dim_operate"(milliseconds to wait=u32 1000) -> ()  [unwired: 1 out]
    }
    frame #1 {
      # "Front Panel Indicators"
      # "Arrange references to all monitor-value related buttons into an array."
      n3 = control-ref of="InjTunnel_Mon"() -> (w49:refnum<vi>)
      n4 = control-ref of="RetDisk1_Mon"() -> (w39:refnum<vi>)
      n5 = control-ref of="RetDisk2_Mon"() -> (w38:refnum<vi>)
      n6 = control-ref of="CoolWedge1_Mon"() -> (w37:refnum<vi>)
      n7 = control-ref of="CoolWedge2_Mon"() -> (w35:refnum<vi>)
      n8 = control-ref of="DCCool_Mon"() -> (w36:refnum<vi>)
      n9 = control-ref of="FreqCool_Mon"() -> (w34:refnum<vi>)
      n10 = control-ref of="AmpCool_Mon"() -> (w33:refnum<vi>)
      n11 = control-ref of="EndCool_Mon"() -> (w32:refnum<vi>)
      n12 = control-ref of="MicWedge1_Mon"() -> (w31:refnum<vi>)
      n13 = control-ref of="MicWedge2_Mon"() -> (w30:refnum<vi>)
      n14 = control-ref of="Thermocouple2_Mon"() -> (w48:refnum<vi>)
      n15 = control-ref of="Thermocouple1_Mon"() -> (w47:refnum<vi>)
      n16 = control-ref of="DCMicro_Mon"() -> (w27:refnum<vi>)
      n17 = control-ref of="AmpMicro_Mon"() -> (w24:refnum<vi>)
      n18 = control-ref of="PhaseMicro_Mon"() -> (w23:refnum<vi>)
      n19 = control-ref of="StartBun_Mon"() -> (w29:refnum<vi>)
      n20 = control-ref of="DCBun_Mon"() -> (w28:refnum<vi>)
      n21 = control-ref of="AmpBun_Mon"() -> (w26:refnum<vi>)
      n22 = control-ref of="PhaseBun_Mon"() -> (w25:refnum<vi>)
      n23 = control-ref of="Trap1Eject_Mon"() -> (w22:refnum<vi>)
      n24 = control-ref of="Trap1Cool_Mon"() -> (w21:refnum<vi>)
      n25 = control-ref of="Trap2Eject_Mon"() -> (w20:refnum<vi>)
      n26 = control-ref of="Trap2Cool_Mon"() -> (w19:refnum<vi>)
      n27 = control-ref of="Trap3Eject_Mon"() -> (w17:refnum<vi>)
      n28 = control-ref of="Trap3Cool_Mon"() -> (w18:refnum<vi>)
      n29 = control-ref of="Thermocouple4_Mon"() -> (w46:refnum<vi>)
      n30 = control-ref of="Thermocouple3_Mon"() -> (w45:refnum<vi>)
      n31 = control-ref of="Trap4Eject_Mon"() -> (w16:refnum<vi>)
      n32 = control-ref of="Trap4Cool_Mon"() -> (w15:refnum<vi>)
      n33 = control-ref of="Trap5Eject_Mon"() -> (w14:refnum<vi>)
      n34 = control-ref of="Trap5Cool_Mon"() -> (w13:refnum<vi>)
      n35 = control-ref of="Trap6Eject_Mon"() -> (w12:refnum<vi>)
      n36 = control-ref of="Trap6Cool_Mon"() -> (w11:refnum<vi>)
      n37 = control-ref of="Trap7Eject_Mon"() -> (w10:refnum<vi>)
      n38 = control-ref of="Trap7Cool_Mon"() -> (w9:refnum<vi>)
      n39 = control-ref of="ExBun1Eject_Mon"() -> (w8:refnum<vi>)
      n40 = control-ref of="ExBun1Cool_Mon"() -> (w7:refnum<vi>)
      n41 = Build Array(w49, w39, w38, w37, w35, w36, w34, w33, w32, w31, w30, w48, w47, w27, w24, w23, w29, w28, w26, w25, w22, w21, w20, w19, w17, w18, w46, w45) -> (w44:refnum<vi>[])
      n42 = control-ref of="ExBun2_Mon"() -> (w6:refnum<vi>)
      n43 = control-ref of="DefLens_Mon"() -> (w5:refnum<vi>)
      n44 = control-ref of="TranTube_Mon"() -> (w4:refnum<vi>)
      n45 = control-ref of="BunLens_Mon"() -> (w40:refnum<vi>)
      n46 = control-ref of="BunDefX_Mon"() -> (w43:refnum<vi>)
      n47 = control-ref of="BunDefY_Mon"() -> (w42:refnum<vi>)
      n48 = control-ref of="CoolPress_Mon"() -> (w3:refnum<vi>)
      n49 = Build Array (concatenate)(w44, w16, w15, w14, w13, w12, w11, w10, w9, w8, w7, w6, w5, w4, w40, w43, w42, w3) -> (w41:refnum<vi>[])
      n50 = for "InitializeIndicators" {
        tunnel: w41 -> [w51] mode=indexing
        n51 = property class="DigNum (strict)"(reference=w51, "Label.BG Color"=u32 16448250 ("Color Box")) -> ()  [unwired: 1 in, 2 out]
      }
    }
    frame #2 {
      # "Pop-up Controllers"
      n52 = control-ref of="RetDisk2"() -> (w88:refnum<vi>)
      n53 = control-ref of="Trap2Cool"() -> (w87:refnum<vi>)
      n54 = control-ref of="ExBun1Cool"() -> (w86:refnum<vi>)
      n55 = control-ref of="CoolWedge1"() -> (w85:refnum<vi>)
      n56 = control-ref of="CoolWedge2"() -> (w84:refnum<vi>)
      n57 = control-ref of="Trap3Cool"() -> (w83:refnum<vi>)
      n58 = control-ref of="Trap5Cool"() -> (w82:refnum<vi>)
      n59 = control-ref of="Trap6Cool"() -> (w81:refnum<vi>)
      n60 = control-ref of="InjTunnel"() -> (w80:refnum<vi>)
      n61 = control-ref of="ExBun2"() -> (w79:refnum<vi>)
      n62 = control-ref of="ExBun1Eject"() -> (w78:refnum<vi>)
      n63 = control-ref of="MicWedge2"() -> (w77:refnum<vi>)
      n64 = control-ref of="Trap4Eject"() -> (w76:refnum<vi>)
      n65 = control-ref of="TranTube"() -> (w75:refnum<vi>)
      n66 = control-ref of="RetDisk1"() -> (w74:refnum<vi>)
      n67 = control-ref of="Trap1Eject"() -> (w73:refnum<vi>)
      n68 = control-ref of="Trap7Cool"() -> (w72:refnum<vi>)
      n69 = control-ref of="AmpCool"() -> (w54:refnum<vi>)
      n70 = control-ref of="AmpBun"() -> (w53:refnum<vi>)
      n71 = Build Array(w88, w87, w86, w85, w84, w83, w82, w81, w80, w79, w78, w77, w76, w75, w74, w73, w72, w54, w53) -> (w57:refnum<vi>[])
      n72 = control-ref of="Trap2Eject"() -> (w71:refnum<vi>)
      n73 = control-ref of="Trap7Eject"() -> (w70:refnum<vi>)
      n74 = control-ref of="BunLens"() -> (w69:refnum<vi>)
      n75 = control-ref of="StartBun"() -> (w68:refnum<vi>)
      n76 = control-ref of="DefLens"() -> (w67:refnum<vi>)
      n77 = control-ref of="Trap3Eject"() -> (w66:refnum<vi>)
      n78 = control-ref of="EndCool"() -> (w65:refnum<vi>)
      n79 = control-ref of="Trap5Eject"() -> (w64:refnum<vi>)
      n80 = control-ref of="Trap6Eject"() -> (w63:refnum<vi>)
      n81 = control-ref of="Trap1Cool"() -> (w62:refnum<vi>)
      n82 = control-ref of="BunDefX"() -> (w61:refnum<vi>)
      n83 = control-ref of="BunDefY"() -> (w60:refnum<vi>)
      n84 = control-ref of="Trap4Cool"() -> (w59:refnum<vi>)
      n85 = control-ref of="MicWedge1"() -> (w58:refnum<vi>)
      n86 = control-ref of="CoolPress"() -> (w55:refnum<vi>)
      n87 = control-ref of="AmpMicro"() -> (w52:refnum<vi>)
      n88 = Build Array (concatenate)(w57, w71, w70, w69, w68, w67, w66, w65, w64, w63, w62, w61, w60, w59, w58, w55, w52) -> (w56:refnum<vi>[])
      n89 = for "Initialize Pop-up to Default" {
        tunnel: w56 -> [w89] mode=indexing
        n90 = invoke class="Bool" method="Reinit To Default"(reference=w89) -> ()  [unwired: 2 in, 3 out]
      }
    }
    frame #3 {
      # "DIM Monitor Values Variables"
      # "Arrange references to all monitor-value related buttons into an array."
      n91 = control-ref of="DCMicro_MonData"() -> (w118:refnum<vi>)
      n92 = control-ref of="CoolPress_MonData"() -> (w91:refnum<vi>)
      n93 = control-ref of="bunBase_MonData"() -> (w92:refnum<vi>)
      n94 = control-ref of="Thermocouple1_MonData"() -> (w124:refnum<vi>)
      n95 = control-ref of="Thermocouple2_MonData"() -> (w125:refnum<vi>)
      n96 = control-ref of="RetDisk1_MonData"() -> (w131:refnum<vi>)
      n97 = control-ref of="RetDisk2_MonData"() -> (w130:refnum<vi>)
      n98 = control-ref of="InjTunnel_MonData"() -> (w139:refnum<vi>)
      n99 = control-ref of="CoolWedge1_MonData"() -> (w138:refnum<vi>)
      n100 = control-ref of="CoolWedge2_MonData"() -> (w137:refnum<vi>)
      n101 = control-ref of="EndCool_MonData"() -> (w136:refnum<vi>)
      n102 = control-ref of="DCCool_MonData"() -> (w135:refnum<vi>)
      n103 = control-ref of="AmpCool_MonData"() -> (w134:refnum<vi>)
      n104 = control-ref of="FreqCool_MonData"() -> (w133:refnum<vi>)
      n105 = control-ref of="MicWedge1_MonData"() -> (w132:refnum<vi>)
      n106 = control-ref of="MicWedge2_MonData"() -> (w120:refnum<vi>)
      n107 = control-ref of="StartBun_MonData"() -> (w119:refnum<vi>)
      n108 = Build Array(w91, w92, w124, w125, w131, w130, w139, w138, w137, w136, w135, w134, w133, w132, w120, w119, w118) -> (w117:refnum<vi>[])
      n109 = control-ref of="AmpMicro_MonData"() -> (w129:refnum<vi>)
      n110 = control-ref of="PhaseMicro_MonData"() -> (w128:refnum<vi>)
      n111 = control-ref of="DCBun_MonData"() -> (w127:refnum<vi>)
      n112 = control-ref of="AmpBun_MonData"() -> (w126:refnum<vi>)
      n113 = control-ref of="PhaseBun_MonData"() -> (w123:refnum<vi>)
      n114 = control-ref of="ExBun2_MonData"() -> (w122:refnum<vi>)
      n115 = control-ref of="TranTube_MonData"() -> (w121:refnum<vi>)
      n116 = control-ref of="DefLens_MonData"() -> (w116:refnum<vi>)
      n117 = control-ref of="BunLens_MonData"() -> (w115:refnum<vi>)
      n118 = control-ref of="Thermocouple3_MonData"() -> (w102:refnum<vi>)
      n119 = Build Array (concatenate)(w117, w129, w128, w127, w126, w123, w122, w121, w116, w115, w102) -> (w114:refnum<vi>[])
      n120 = control-ref of="Trap4Cool_MonData"() -> (w101:refnum<vi>)
      n121 = control-ref of="Trap5Cool_MonData"() -> (w100:refnum<vi>)
      n122 = control-ref of="Thermocouple4_MonData"() -> (w113:refnum<vi>)
      n123 = control-ref of="BunDefX_MonData"() -> (w112:refnum<vi>)
      n124 = control-ref of="BunDefY_MonData"() -> (w111:refnum<vi>)
      n125 = control-ref of="Trap1Cool_MonData"() -> (w110:refnum<vi>)
      n126 = control-ref of="Trap2Cool_MonData"() -> (w109:refnum<vi>)
      n127 = control-ref of="Trap3Cool_MonData"() -> (w108:refnum<vi>)
      n128 = control-ref of="Trap6Cool_MonData"() -> (w99:refnum<vi>)
      n129 = Build Array (concatenate)(w114, w113, w112, w111, w110, w109, w108, w101, w100, w99) -> (w95:refnum<vi>[])
      n130 = control-ref of="ExBun1Eject_MonData"() -> (w94:refnum<vi>)
      n131 = control-ref of="ExBun1Cool_MonData"() -> (w93:refnum<vi>)
      n132 = control-ref of="Trap7Cool_MonData"() -> (w107:refnum<vi>)
      n133 = control-ref of="Trap1Eject_MonData"() -> (w106:refnum<vi>)
      n134 = control-ref of="Trap2Eject_MonData"() -> (w105:refnum<vi>)
      n135 = control-ref of="Trap3Eject_MonData"() -> (w104:refnum<vi>)
      n136 = control-ref of="Trap4Eject_MonData"() -> (w103:refnum<vi>)
      n137 = control-ref of="Trap5Eject_MonData"() -> (w98:refnum<vi>)
      n138 = control-ref of="Trap6Eject_MonData"() -> (w97:refnum<vi>)
      n139 = control-ref of="Trap7Eject_MonData"() -> (w96:refnum<vi>)
      n140 = Build Array (concatenate)(w95, w94, w93, w107, w106, w105, w104, w103, w98, w97, w96) -> (w90:refnum<vi>[])
      n141 = for "Subscribe to DIM Monitor Values" {
        tunnel: w90 -> [w140] mode=indexing
        n142 = property class="Clust (strict)"(reference=w140) -> ("Label.Text"=w142:string)  [unwired: 1 in, 2 out]
        n143 = Match Pattern(string=w142, regular expression="Data") -> (before substring=w141:string)  [unwired: 1 in, 3 out]
        n144 = call "DimIndicators.dic_info_service.vi"("controlRef"=w140, "serviceName"=w141) -> ()  [unwired: 16 in, 2 out]
      }
    }
    frame #4 {
      # "DIM Set Values Variables"
      n145 = control-ref of="bunBase_SetData"() -> (w167:refnum<vi>)
      n146 = control-ref of="RetDisk1_SetData"() -> (w168:refnum<vi>)
      n147 = control-ref of="RetDisk2_SetData"() -> (w169:refnum<vi>)
      n148 = control-ref of="InjTunnel_SetData"() -> (w187:refnum<vi>)
      n149 = control-ref of="CoolWedge1_SetData"() -> (w186:refnum<vi>)
      n150 = control-ref of="CoolWedge2_SetData"() -> (w185:refnum<vi>)
      n151 = control-ref of="EndCool_SetData"() -> (w184:refnum<vi>)
      n152 = control-ref of="DCCool_SetData"() -> (w183:refnum<vi>)
      n153 = control-ref of="AmpCool_SetData"() -> (w182:refnum<vi>)
      n154 = control-ref of="FreqCool_SetData"() -> (w181:refnum<vi>)
      n155 = control-ref of="MicWedge1_SetData"() -> (w180:refnum<vi>)
      n156 = control-ref of="MicWedge2_SetData"() -> (w179:refnum<vi>)
      n157 = control-ref of="StartBun_SetData"() -> (w178:refnum<vi>)
      n158 = control-ref of="DCMicro_SetData"() -> (w177:refnum<vi>)
      n159 = control-ref of="CoolPress_SetData"() -> (w146:refnum<vi>)
      n160 = control-ref of="AmpMicro_SetData"() -> (w166:refnum<vi>)
      n161 = control-ref of="PhaseMicro_SetData"() -> (w165:refnum<vi>)
      n162 = control-ref of="PercentNeon_SetData"() -> (w144:refnum<vi>)
      n163 = control-ref of="BunDefY_SetData"() -> (w147:refnum<vi>)
      n164 = control-ref of="DCBun_SetData"() -> (w164:refnum<vi>)
      n165 = control-ref of="AmpBun_SetData"() -> (w176:refnum<vi>)
      n166 = control-ref of="PhaseBun_SetData"() -> (w175:refnum<vi>)
      n167 = control-ref of="ExBun2_SetData"() -> (w174:refnum<vi>)
      n168 = control-ref of="TranTube_SetData"() -> (w173:refnum<vi>)
      n169 = control-ref of="DefLens_SetData"() -> (w172:refnum<vi>)
      n170 = control-ref of="BunLens_SetData"() -> (w171:refnum<vi>)
      n171 = control-ref of="BunDefX_SetData"() -> (w170:refnum<vi>)
      n172 = control-ref of="Trap1Cool_SetData"() -> (w148:refnum<vi>)
      n173 = control-ref of="Trap2Cool_SetData"() -> (w149:refnum<vi>)
      n174 = control-ref of="Trap3Cool_SetData"() -> (w150:refnum<vi>)
      n175 = control-ref of="Trap4Cool_SetData"() -> (w163:refnum<vi>)
      n176 = control-ref of="Trap5Cool_SetData"() -> (w162:refnum<vi>)
      n177 = control-ref of="Trap6Cool_SetData"() -> (w161:refnum<vi>)
      n178 = control-ref of="Trap7Cool_SetData"() -> (w160:refnum<vi>)
      n179 = control-ref of="Trap1Eject_SetData"() -> (w159:refnum<vi>)
      n180 = control-ref of="Trap2Eject_SetData"() -> (w158:refnum<vi>)
      n181 = control-ref of="Trap5Eject_SetData"() -> (w155:refnum<vi>)
      n182 = control-ref of="Trap7Eject_SetData"() -> (w153:refnum<vi>)
      n183 = control-ref of="ExBun1Cool_SetData"() -> (w151:refnum<vi>)
      n184 = control-ref of="Trap4Eject_SetData"() -> (w156:refnum<vi>)
      n185 = control-ref of="Trap6Eject_SetData"() -> (w154:refnum<vi>)
      n186 = control-ref of="ExBun1Eject_SetData"() -> (w152:refnum<vi>)
      n187 = control-ref of="Trap3Eject_SetData"() -> (w157:refnum<vi>)
      n188 = Build Array(w144, w146, w167, w168, w169, w187, w186, w185, w184, w183, w182, w181, w180, w179, w178, w177, w166, w165, w164, w176, w175, w174, w173, w172, w171, w170, w147, w148, w149, w150, w163, w162, w161, w160, w159, w158, w157, w156, w155, w154, w153, w152, w151) -> (w145:refnum<vi>[])
      n189 = for "Subscribe to DIM Set Values" {
        tunnel: w145 -> [w188] mode=indexing
        tunnel: w145 -> [w192] mode=indexing
        n190 = property class="Clust (strict)"(reference=w188) -> ("Label.Text"=w191:string)  [unwired: 1 in, 2 out]
        n191 = Match Pattern(string=w191, regular expression="Data") -> (before substring=w189:string)  [unwired: 1 in, 3 out]
        n192 = call "DimIndicators.dic_info_service.vi"("controlRef"=w192, "serviceName"=w189) -> ()  [unwired: 16 in, 2 out]
      }
    }
    frame #5 {
      # "DIM Set Value Info Variables"
      n193 = control-ref of="CoolPress_SetValueInfoData"() -> (w199:refnum<vi>)
      n194 = control-ref of="bunBase_SetValueInfoData"() -> (w220:refnum<vi>)
      n195 = control-ref of="RetDisk1_SetValueInfoData"() -> (w219:refnum<vi>)
      n196 = control-ref of="RetDisk2_SetValueInfoData"() -> (w237:refnum<vi>)
      n197 = control-ref of="InjTunnel_SetValueInfoData"() -> (w236:refnum<vi>)
      n198 = control-ref of="CoolWedge1_SetValueInfoData"() -> (w235:refnum<vi>)
      n199 = control-ref of="CoolWedge2_SetValueInfoData"() -> (w234:refnum<vi>)
      n200 = control-ref of="EndCool_SetValueInfoData"() -> (w233:refnum<vi>)
      n201 = control-ref of="DCCool_SetValueInfoData"() -> (w232:refnum<vi>)
      n202 = control-ref of="AmpCool_SetValueInfoData"() -> (w231:refnum<vi>)
      n203 = control-ref of="FreqCool_SetValueInfoData"() -> (w230:refnum<vi>)
      n204 = control-ref of="MicWedge1_SetValueInfoData"() -> (w229:refnum<vi>)
      n205 = control-ref of="MicWedge2_SetValueInfoData"() -> (w228:refnum<vi>)
      n206 = control-ref of="StartBun_SetValueInfoData"() -> (w227:refnum<vi>)
      n207 = control-ref of="DCMicro_SetValueInfoData"() -> (w218:refnum<vi>)
      n208 = control-ref of="AmpMicro_SetValueInfoData"() -> (w217:refnum<vi>)
      n209 = control-ref of="PhaseMicro_SetValueInfoData"() -> (w216:refnum<vi>)
      n210 = control-ref of="BunDefY_SetValueInfoData"() -> (w196:refnum<vi>)
      n211 = control-ref of="BunDefX_SetValueInfoData"() -> (w195:refnum<vi>)
      n212 = control-ref of="Trap1Cool_SetValueInfoData"() -> (w215:refnum<vi>)
      n213 = control-ref of="DCBun_SetValueInfoData"() -> (w197:refnum<vi>)
      n214 = control-ref of="AmpBun_SetValueInfoData"() -> (w226:refnum<vi>)
      n215 = control-ref of="PhaseBun_SetValueInfoData"() -> (w225:refnum<vi>)
      n216 = control-ref of="ExBun2_SetValueInfoData"() -> (w224:refnum<vi>)
      n217 = control-ref of="Trap3Cool_SetValueInfoData"() -> (w213:refnum<vi>)
      n218 = control-ref of="DefLens_SetValueInfoData"() -> (w222:refnum<vi>)
      n219 = control-ref of="Trap2Cool_SetValueInfoData"() -> (w214:refnum<vi>)
      n220 = control-ref of="Trap4Cool_SetValueInfoData"() -> (w212:refnum<vi>)
      n221 = control-ref of="ExBun1Eject_SetValueInfoData"() -> (w201:refnum<vi>)
      n222 = control-ref of="TranTube_SetValueInfoData"() -> (w223:refnum<vi>)
      n223 = control-ref of="BunLens_SetValueInfoData"() -> (w221:refnum<vi>)
      n224 = control-ref of="ExBun1Cool_SetValueInfoData"() -> (w200:refnum<vi>)
      n225 = control-ref of="bunBase_SetValueInfoData"() -> (w194:refnum<vi>)
      n226 = control-ref of="Trap5Cool_SetValueInfoData"() -> (w211:refnum<vi>)
      n227 = control-ref of="Trap1Eject_SetValueInfoData"() -> (w208:refnum<vi>)
      n228 = control-ref of="Trap5Eject_SetValueInfoData"() -> (w204:refnum<vi>)
      n229 = control-ref of="Trap6Cool_SetValueInfoData"() -> (w210:refnum<vi>)
      n230 = control-ref of="Trap7Cool_SetValueInfoData"() -> (w209:refnum<vi>)
      n231 = control-ref of="Trap2Eject_SetValueInfoData"() -> (w207:refnum<vi>)
      n232 = control-ref of="Trap6Eject_SetValueInfoData"() -> (w203:refnum<vi>)
      n233 = control-ref of="Trap3Eject_SetValueInfoData"() -> (w206:refnum<vi>)
      n234 = control-ref of="Trap4Eject_SetValueInfoData"() -> (w205:refnum<vi>)
      n235 = control-ref of="Trap7Eject_SetValueInfoData"() -> (w202:refnum<vi>)
      n236 = control-ref of="PercentNeon_SetValueInfoData"() -> (w193:refnum<vi>)
      n237 = Build Array(w193, w194, w195, w199, w220, w219, w237, w236, w235, w234, w233, w232, w231, w230, w229, w228, w227, w218, w217, w216, w196, w197, w226, w225, w224, w223, w222, w221, w215, w214, w213, w212, w201, w200, w211, w210, w209, w208, w207, w206, w205, w204, w203, w202) -> (w198:refnum<vi>[])
      n238 = for "Subscribe to DIM Set Info Value" {
        tunnel: w198 -> [w238] mode=indexing
        tunnel: w198 -> [w242] mode=indexing
        n239 = property class="Clust (strict)"(reference=w238) -> ("Label.Text"=w241:string)  [unwired: 1 in, 2 out]
        n240 = Match Pattern(string=w241, regular expression="Data") -> (before substring=w239:string)  [unwired: 1 in, 3 out]
        n241 = call "DimIndicators.dic_info_service.vi"("controlRef"=w242, "serviceName"=w239) -> ()  [unwired: 16 in, 2 out]
      }
    }
    frame #6 {
      # "Create Dim Last Loaded File Variable"
      # "Sort Variables"
      n242 = call "SortArraysPLC.vi"("Pop-up Con."=w257, "FPIndicator in"=w258, "DIMControlMon"=w256, "DIMControSet"=w255, "SetValueInfo"=w254) -> ("Pop-up Con. out"=w249:refnum<vi>[], "FPIndicator out"=w250:refnum<vi>[], "DIMControlMon out"=w251:refnum<vi>[], "DIMControSet out"=w252:refnum<vi>[], "SetValueInfo out"=w253:refnum<vi>[])  [unwired: 18 in]
      n243 = control-ref of="ListOfBases_Data"() -> (w244:refnum<vi>)
      n244 = control-ref of="SetFileLocation_Data"() -> (w245:refnum<vi>)
      n245 = control-ref of="Last Loaded File_Data"() -> (w247:refnum<vi>)
      n246 = call "DimIndicators.dic_info_service.vi"("controlRef"=w244, "serviceName"="ListOfBases" ("string")) -> ()  [unwired: 16 in, 2 out]
      n247 = call "DimIndicators.dic_info_service.vi"("controlRef"=w247, "serviceName"="bun" ("string")) -> ()  [unwired: 16 in, 2 out]
      n248 = call "DimIndicators.dic_info_service.vi"("controlRef"=w245, "serviceName"="SetFileLocation" ("string")) -> ()  [unwired: 16 in, 2 out]
    }
    frame #7 {
      # "Create sub-panel\narray"
      n249 = Array Size(array=w259) -> (size(s)=w263:i32)
      n250 = Initialize Array(refnum<vi> refnum ("vi reference"), w263) -> (w266:refnum<vi>[])
      n251 = while "Wait For User Commands and Variable Changes" {
        tunnel: w267 -> [w275]
        tunnel: w264 -> [w274]
        shift-right: [w272] -> w262
        shift-left: w266 -> [w273]
        tunnel: w261 -> [w268]
        tunnel: w260 -> [w269]
        tunnel: w259 -> [w270]
        stop <- w276 stop-if-true
        n252 = event "Decifier User Selection or  Variable Changes" shown="[0] Menu Selection (User)" {
          selector: _ -> [_ _ _ _ _ _ _ _ _ _ _ _ _]
          dyn-events: _ -> [_ _ _ _ _ _ _ _ _ _ _ _ _]
          timeout: -1 -> [_ _ _ _ _ _ _ _ _ _ _ _ _]
          tunnel: [w278 _ _ _ _ _ _ _ _ _ _ _ TRUE ("stop")] -> w276
          tunnel: w275 -> [_ _ _ _ _ _ w465 _ _ _ _ _ w534]
          tunnel: w274 -> [_ _ _ _ _ _ w464 w484 _ _ _ _ _]
          tunnel: w273 -> [w281 w355 w389 w396 w421 w432 w468 w483 w511 w519 w526 w532 w533]
          tunnel: [w281 w355 w389 w396 w421 w432 w468 w483 w511 w517 w524 w532 _] -> w272
          tunnel: w268 -> [w279 w354 w384 w397 _ w431 _ _ w509 _ _ _ w535]
          tunnel: w269 -> [w277 w353 w383 w398 _ _ _ _ _ _ _ _ w536]
          tunnel: w270 -> [_ _ _ _ _ _ _ _ _ w513 _ _ _]
          event Menu Selection (User) {
            # "Deal With Menu Selections"
            n253 = event-data() -> ("ItemTag"=w280:string)  [unwired: 1 in]
            n254 = case "Selection?" shown="\"BUNAPP_FILE_SAVE\"" w280 {
              tunnel: w279 -> [_ w286 w306 w346 _ _]
              tunnel: [_ _ _ _ _ TRUE ("stop")] -> w278
              tunnel: w277 -> [_ w282 w301 w333 _ _]
              frame "False", Default {
              }
              frame "BUNAPP_FILE_SAVE" {
                # "Save Loaded Voltages to a File"
                n255 = property on="SetFileLocation" class="Path"() -> ("Value"=w287:path)  [unwired: 2 in, 2 out]
                n256 = call "SaveLoadedValues.vi"("Panel Location?"=w287, "DIMControlSet in"=w286) -> ("File Saved?"=w288:bool, "File Name"=w285:string, "DIMControlSet out"=w283:refnum<vi>[], "Path"=w284:path)  [unwired: 14 in]
                n257 = case "Accepted?" shown="True" w288 {
                  tunnel: w285 -> [_ w298]
                  tunnel: "bun" ("string") -> [_ w300]
                  tunnel: w283 -> [_ w299]
                  tunnel: w284 -> [_ w297]
                  tunnel: w282 -> [_ w291]
                  frame False {
                  }
                  frame True {
                    n258 = call "UpdateLastLoadedFile.vi"("LoadOrSave"=enum16{"Load", "Save"}."Save", "GUIName"=w300, "FileNameIn"=w298) -> ()  [unwired: 13 in]
                    n259 = call "PrepareSignals.vi"("SetValueInfo in"=w291, "setfile path"=w297, "Enum"=enum16{"Save", "Load"}."Save", "DIMControSet in"=w299) -> ("indexed loaded Array"=w295:dbl[][], "Name Array"=w296:string[], "DIMControSet out"=w294:refnum<vi>[])  [unwired: 5 in]
                    n260 = call "CompareArrays.vi"("indexed loaded Array"=w295, "Name Array"=w296, "DIMControSet"=w294) -> ("Table for loading values"=w293:string[][])  [unwired: 4 in]
                    n261 = call "LoadSetFileToDIM.vi"("output array"=w293) -> ()  [unwired: 2 in]
                  }
                }
              }
              frame "BUNAPP_FILE_LOAD" {
                # "Promt User For File to Load"
                n262 = property on="SetFileLocation" class="Path"() -> ("Value"=w303:path)  [unwired: 2 in, 2 out]
                n263 = File Dialog(6:"*.set" ("pattern (all files)"), 11:w303) -> (0:w302:errorcluster, 1:w307:bool, 3:w304:path)  [unwired: 5 in, 1 out]
                n264 = case shown="No Error" w302 {
                  tunnel: w307 -> [w312 w330]
                  tunnel: w306 -> [w311 _]
                  tunnel: w304 -> [w309 _]
                  tunnel: w301 -> [w308 _]
                  frame No Error {
                    n265 = Strip Path(path=w309) -> (name=w310:string)  [unwired: 1 out]
                    n266 = case "Load File?" shown="False" w312 {
                      tunnel: w311 -> [w326 _]
                      tunnel: w310 -> [w320 _]
                      tunnel: w309 -> [w321 _]
                      tunnel: w308 -> [w314 _]
                      frame False {
                        n267 = control-ref of="ListOfBases_Data"() -> (w313:refnum<vi>)
                        n268 = call "PrepareSignals.vi"("ListOfBases_Data"=w313, "SetValueInfo in"=w314, "setfile path"=w321, "Enum"=enum16{"Save", "Load"}."Load", "Display Message to \nUser"=TRUE ("Display Message to \nUser"), "DIMControSet in"=w326) -> ("indexed loaded Array"=w324:dbl[][], "Name Array"=w323:string[], "DIMControSet out"=w325:refnum<vi>[])  [unwired: 3 in]
                        n269 = call "CompareArrays.vi"("indexed loaded Array"=w324, "Name Array"=w323, "DIMControSet"=w325) -> ("Table for loading values"=w322:string[][])  [unwired: 4 in]
                        n270 = call "LoadSet.vi"("File Name In"=w320, "output array"=w322) -> ("File Name out"=w319:string, "Accepted"=w318:bool)  [unwired: 8 in]
                        n271 = case "Accepted?" shown="True" w318 {
                          tunnel: w319 -> [_ w329]
                          tunnel: "bun" ("string") -> [_ w328]
                          frame False {
                          }
                          frame True {
                            n272 = call "UpdateLastLoadedFile.vi"("LoadOrSave"=enum16{"Load", "Save"}."Load", "GUIName"=w328, "FileNameIn"=w329) -> ()  [unwired: 13 in]
                          }
                        }
                      }
                      frame True {
                      }
                    }
                  }
                  frame Error {
                    n273 = Not(x=w330) -> (.not. x?=w331:bool)
                    n274 = call "Display Message to User"("Enable"=w331) -> ()  [unwired: 9 in, 2 out]
                  }
                }
              }
              frame "BUNAPP_FILE_ZERO" {
                w337 = "All Signals Go To Zero.set" ("File Name")
                # "Set Voltages to Zero"
                n275 = property on="SetFileLocation" class="Path"() -> ("Value"=w335:path)  [unwired: 2 in, 2 out]
                n276 = Build Path(base path=w335, name or relative path=w337) -> (appended path=w336:path)
                n277 = control-ref of="ListOfBases_Data"() -> (w332:refnum<vi>)
                n278 = call "PrepareSignals.vi"("ListOfBases_Data"=w332, "SetValueInfo in"=w333, "setfile path"=w336, "Enum"=enum16{"Save", "Load"}."Load", "Display Message to \nUser"=TRUE ("Display Message to \nUser"), "DIMControSet in"=w346) -> ("indexed loaded Array"=w344:dbl[][], "Name Array"=w343:string[], "DIMControSet out"=w345:refnum<vi>[])  [unwired: 3 in]
                n279 = call "CompareArrays.vi"("indexed loaded Array"=w344, "Name Array"=w343, "DIMControSet"=w345) -> ("Table for loading values"=w342:string[][])  [unwired: 4 in]
                n280 = call "LoadSet.vi"("File Name In"=w337, "output array"=w342) -> ("File Name out"=w340:string, "Accepted"=w341:bool)  [unwired: 8 in]
                n281 = case "Accepted?" shown="True" w341 {
                  tunnel: w340 -> [_ w349]
                  tunnel: "bun" ("string") -> [_ w348]
                  frame False {
                  }
                  frame True {
                    n282 = call "UpdateLastLoadedFile.vi"("LoadOrSave"=enum16{"Load", "Save"}."Load", "GUIName"=w348, "FileNameIn"=w349) -> ()  [unwired: 13 in]
                  }
                }
              }
              frame "Legend" {
                # "Open Legend"
                n283 = call "Legend.vi"("i ref in"=refnum<vi> refnum) -> ("i ref out"=→"i ref out":refnum<vi>)  [unwired: 10 in]
              }
              frame "BUNAPP_FILE_EXIT" {
                # "Exit"
              }
            }
          }
          event Value Change {
            n284 = event-data() -> ("NewVal"=w356:T1)  [unwired: 1 in]
            n285 = stacked-sequence {
              tunnel: w356 -> [w359 _]
              tunnel: w354 -> [_ w376]
              tunnel: w353 -> [_ w375]
              frame #0 {
                # "Update Set File Location"
                n286 = Unbundle By Name(w359) -> ("data"=w367:string, "no link"=w366:bool, "quality"=w365:i32)
                n287 = case "Link?" shown="False" w366 {
                  tunnel: w365 -> [w371 _]
                  tunnel: [w370 UtilityLib.valueStatus."no info available" ("valueStatus")] -> w368
                  tunnel: w367 -> [w369 _]
                  tunnel: [w369 w372] -> w363
                  frame False {
                    n288 = call "CoreLib.quality 2 status.vi"("quality"=w371) -> ("valueStatus"=w370:T7)  [unwired: 18 in]
                  }
                  frame True {
                    n289 = call "EmptyString.vi"() -> ("String"=w372:string)
                  }
                }
                n290 = Type Cast(type="" ("regular expression"), x=w363) -> (*(type *) &x=w362:string)
                n291 = String To Path(string=w362) -> (path=w358:path)
                n292 = control-ref of="SetFileLocation"() -> (w357:refnum<vi>)
                n293 = Build Path(base path=w358, name or relative path="bunControl") -> (appended path=w360:path)
                n294 = property class="Path"(reference=w357, "Value"=w360) -> ()  [unwired: 1 in, 2 out]
                n295 = call "UtilityLib.set color of GUI object.vi"("GUI object Ref"=w357, "valueStatus"=w368) -> ()  [unwired: 17 in, 1 out]
              }
              frame #1 {
                # "Update Last Loaded File"
                n296 = control-ref of="SetFileLocation"() -> (w380:refnum<vi>)
                n297 = control-ref of="Last Loaded File"() -> (w381:refnum<vi>)
                n298 = control-ref of="Last Loaded File_Data"() -> (w379:refnum<vi>)
                n299 = control-ref of="ListOfBases_Data"() -> (w374:refnum<vi>)
                n300 = property class="Clust (strict)"(reference=w379) -> ("Value"=w378:T8)  [unwired: 1 in, 2 out]
                n301 = call "LastLoadedFile.vi"("SetFileLocation"=w380, "Last Loaded File"=w381, "GUIName"="bun", "DIMControSet in"=w376, "SetValueInfo in"=w375, "NewVal"=w378, "ListOfBases_Data"=w374) -> ()  [unwired: 13 in]
              }
            }
          }
          event Value Change {
            # "Update Last Loaded File"
            n302 = event-data() -> ("NewVal"=w386:T1)  [unwired: 1 in]
            n303 = control-ref of="SetFileLocation"() -> (w388:refnum<vi>)
            n304 = control-ref of="Last Loaded File"() -> (w387:refnum<vi>)
            n305 = control-ref of="ListOfBases_Data"() -> (w382:refnum<vi>)
            n306 = call "LastLoadedFile.vi"("SetFileLocation"=w388, "Last Loaded File"=w387, "GUIName"="bun", "DIMControSet in"=w384, "SetValueInfo in"=w383, "NewVal"=w386, "ListOfBases_Data"=w382) -> ()  [unwired: 13 in]
          }
          event "bunBase": Value Change {
            w390 = "bunBase" ("string")
            # "Is Base in Range?"
            # "Update  Set Values"
            n307 = event-data() -> ("NewVal"=w393:dbl, "OldVal"=w392:dbl)  [unwired: 1 in, 4 out]
            n308 = control-ref of="ListOfBases_Data"() -> (w391:refnum<vi>)
            n309 = call "IsBaseInRange.vi"("SetValueInfo"=w398, "DIMControSet"=w397, "ListOfBases_Data"=w391, "NewVal in"=w393, "Base Name"=w390) -> ("NewVal Out"=w394:dbl, "In Range"=w395:bool)  [unwired: 13 in]
            n310 = case "Base In Range?" shown="True" w395 {
              tunnel: w394 -> [_ w403]
              tunnel: w392 -> [w399 _]
              tunnel: w390 -> [_ w400]
              frame False {
                n311 = property on="bunBase" class="DigNum (strict)"("Value"=w399) -> ()  [unwired: 2 in, 2 out]
              }
              frame True {
                n312 = call-poly "CoreLib.data 2 byte array.vi"("i16"=i16 1 ("element")) -> ("byteArray out"=w402:T6)  [unwired: 18 in]
                n313 = property on="bunBase" class="DigNum (strict)"("Value"=w403) -> ()  [unwired: 2 in, 2 out]
                n314 = call-poly "CoreLib.data 2 byte array.vi"("byteArray"=w402, "f64"=w403) -> ("byteArray out"=w407:T6)  [unwired: 17 in]
                n315 = Flatten To String(anything=TRUE) -> (data string=w406:string)  [unwired: 3 in, 2 out]
                n316 = Concatenate Strings("SetPLC" ("string"), w400) -> (w412:string)
                n317 = call-poly "CoreLib.data 2 byte array.vi"("byteArray"=w407, "string"=w406) -> ("byteArray out"=w404:T6)  [unwired: 17 in]
                n318 = Bundle By Name(cluster="call cluster in", "Object"="PLC", "Selector"=w412, "CallType"=enum16{"simple", "synchronous", "asynchronous"}."simple", "Data"=w404) -> (w409:T4)
                n319 = call "CoreLib.call process.vi"("call cluster in"=w409) -> ()  [unwired: 13 in, 2 out]
              }
            }
          }
          event "PercentNeon": Value Change {
            # "Get Set Value Info?"
            # "Set Percent Neon"
            n320 = event-data() -> ("NewVal"=w418:dbl, "OldVal"=w415:dbl)  [unwired: 1 in]
            n321 = control-ref of="PercentNeon_SetValueInfoData"() -> (w414:refnum<vi>)
            n322 = property class="Clust (strict)"(reference=w414) -> ("Value"=w420:T9)  [unwired: 1 in, 2 out]
            n323 = Unbundle By Name(w420) -> ("data"=w419:dbl[], "no link"=w417:bool)
            n324 = case "No Link?" shown="False" w417 {
              tunnel: w419 -> [w425 _]
              tunnel: w418 -> [w424 _]
              tunnel: [w423 w426] -> w416
              tunnel: w415 -> [w422 w426]
              frame False {
                n325 = call "SetPercentNeon.vi"("data"=w425, "NewVal"=w424, "Old Value"=w422) -> ("Set Value"=w423:dbl)  [unwired: 16 in]
              }
              frame True {
              }
            }
            n326 = property on="PercentNeon" class="DigNum (strict)"("Value"=w416) -> ()  [unwired: 2 in, 2 out]
          }
          event Value Change {
            # "File Up To Date?"
            n327 = event-data() -> ("CtlRef"=w427:refnum<vi>, "NewVal"=w433:T2)  [unwired: 1 in, 3 out]
            n328 = property class="Clust (strict)"(reference=w427) -> ("Label.Text"=w430:string)  [unwired: 1 in, 2 out]
            n329 = property on="FileUpToDate" class="Bool (strict)"() -> ("Value"=w429:bool)  [unwired: 2 in, 2 out]
            n330 = case shown="\"PercentNeon_SetData\"" w430 {
              tunnel: w433 -> [_ w436 w450]
              frame "False", Default {
              }
              frame "bunBase_SetData" {
                # "Update bunBase Set Value"
                n331 = Unbundle By Name(w436) -> ("data"=w437:dbl[], "no link"=w438:bool, "quality"=w440:i32)
                n332 = case "Link?" shown="False" w438 {
                  tunnel: w440 -> [w442 _]
                  tunnel: [w441 UtilityLib.valueStatus."no info available" ("valueStatus")] -> w439
                  tunnel: w437 -> [w444 _]
                  tunnel: [w443 inf] -> w434
                  frame False {
                    n333 = call "CoreLib.quality 2 status.vi"("quality"=w442) -> ("valueStatus"=w441:T7)  [unwired: 18 in]
                    n334 = Index Array(array=w444, index #1=0 ("index")) -> (element #1=w443:dbl)  [unwired: 1 in, 1 out]
                  }
                  frame True {
                  }
                }
                n335 = control-ref of="bunBase"() -> (w435:refnum<vi>)
                n336 = property on="bunBase" class="DigNum (strict)"("Value"=w434) -> ()  [unwired: 2 in, 2 out]
                n337 = call "UtilityLib.set color of GUI object.vi"("GUI object Ref"=w435, "valueStatus"=w439) -> ()  [unwired: 17 in, 1 out]
              }
              frame "PercentNeon_SetData" {
                # "Update bunBase Set Value"
                n338 = Unbundle By Name(w450) -> ("data"=w451:dbl[], "no link"=w452:bool, "quality"=w454:i32)
                n339 = case "Link?" shown="False" w452 {
                  tunnel: w454 -> [w456 _]
                  tunnel: [w455 UtilityLib.valueStatus."no info available" ("valueStatus")] -> w453
                  tunnel: w451 -> [w458 _]
                  tunnel: [w457 inf] -> w449
                  frame False {
                    n340 = call "CoreLib.quality 2 status.vi"("quality"=w456) -> ("valueStatus"=w455:T7)  [unwired: 18 in]
                    n341 = Index Array(array=w458, index #1=0 ("index")) -> (element #1=w457:dbl)  [unwired: 1 in, 1 out]
                  }
                  frame True {
                  }
                }
                n342 = control-ref of="PercentNeon"() -> (w448:refnum<vi>)
                n343 = property on="PercentNeon" class="DigNum (strict)"("Value"=w449) -> ()  [unwired: 2 in, 2 out]
                n344 = call "UtilityLib.set color of GUI object.vi"("GUI object Ref"=w448, "valueStatus"=w453) -> ()  [unwired: 17 in, 1 out]
              }
            }
            n345 = call "FileUpToDate.vi"("FileUpToDate in"=w429, "DIMControSet out"=w431, "CtlRef"=w427) -> ("FileUpToDate out"=w428:bool)  [unwired: 16 in]
            n346 = property on="FileUpToDate" class="Bool (strict)"("Value"=w428) -> ()  [unwired: 2 in, 2 out]
          }
          event Value Change {
            # "Find Monitor Value Index"
            # "Updating a Monitor Value"
            n347 = event-data() -> ("CtlRef"=w466:refnum<vi>, "NewVal"=w469:T3)  [unwired: 1 in, 4 out]
            n348 = Search 1D Array(1D array=w465, element=w466) -> (index of element=w467:i32)  [unwired: 1 in]
            n349 = Index Array(array=w464, index=w467) -> (element=w462:refnum<vi>)
            n350 = Not A Number/Path/Refnum?(number/path/refnum=w462) -> (NaN/Path/Refnum?=w463:bool)
            n351 = case "Indicator does not exists?" shown="False" w463 {
              tunnel: w469 -> [_ w476]
              tunnel: w462 -> [_ w470]
              frame True {
              }
              frame False {
                n352 = Unbundle By Name(w476) -> ("data"=w472:dbl, "no link"=w473:bool, "quality"=w475:i32)
                n353 = case shown="False" w473 {
                  tunnel: w475 -> [w479 _]
                  tunnel: [w478 UtilityLib.valueStatus."no info available" ("valueStatus")] -> w474
                  tunnel: w472 -> [w477 _]
                  tunnel: [w477 inf] -> w471
                  frame False {
                    n354 = call "CoreLib.quality 2 status.vi"("quality"=w479) -> ("valueStatus"=w478:T7)  [unwired: 18 in]
                  }
                  frame True {
                  }
                }
                n355 = property class="DigNum (strict)"(reference=w470, "Value"=w471) -> ()  [unwired: 1 in, 2 out]
                n356 = call "TextColor.vi"("valueStatus"=w474, "reference"=w470) -> ()  [unwired: 10 in]
              }
            }
          }
          event Value Change {
            n357 = event-data() -> ("CtlRef"=w482:refnum<vi>, "NewVal"=w485:T3)  [unwired: 1 in, 4 out]
            n358 = for "Check if Indicator Exists for the Monitor Value?" {
              tunnel: w485 -> [w494]
              tunnel: w484 -> [w491] mode=indexing
              tunnel: w482 -> [w490]
              # "Updating a Monitor Value"
              n359 = property class="DigNum (strict)"(reference=w491) -> (reference out=w486:refnum<vi>, "Label.Text"=w488:string)  [unwired: 1 in, 1 out]
              n360 = property class="Clust (strict)"(reference=w490) -> ("Label.Text"=w492:string)  [unwired: 1 in, 2 out]
              n361 = Match Pattern(string=w492, regular expression="Data") -> (before substring=w487:string)  [unwired: 1 in, 3 out]
              n362 = Equal?(x=w488, y=w487) -> (x = y?=w489:bool)
              n363 = case "Indicator exists?" shown="True" w489 {
                tunnel: w494 -> [w501 _]
                tunnel: w486 -> [w496 _]
                frame True {
                  n364 = Unbundle By Name(w501) -> ("data"=w498:dbl, "no link"=w499:bool, "quality"=w500:i32)
                  n365 = case shown="False" w499 {
                    tunnel: w500 -> [w504 _]
                    tunnel: [w503 UtilityLib.valueStatus."no info available" ("valueStatus")] -> w495
                    tunnel: w498 -> [w502 _]
                    tunnel: [w502 inf] -> w497
                    frame False {
                      n366 = call "CoreLib.quality 2 status.vi"("quality"=w504) -> ("valueStatus"=w503:T7)  [unwired: 18 in]
                    }
                    frame True {
                    }
                  }
                  n367 = property class="DigNum (strict)"(reference=w496, "Value"=w497) -> ()  [unwired: 1 in, 2 out]
                  n368 = call "TextColor.vi"("valueStatus"=w495, "reference"=w496) -> ()  [unwired: 10 in]
                }
                frame False {
                }
              }
            }
          }
          event Value Change {
            # "File Up To Date?"
            n369 = event-data() -> ("CtlRef"=w507:refnum<vi>)  [unwired: 1 in, 5 out]
            n370 = property on="FileUpToDate" class="Bool (strict)"() -> ("Value"=w508:bool)  [unwired: 2 in, 2 out]
            n371 = call "FileUpToDate.vi"("FileUpToDate in"=w508, "DIMControSet out"=w509, "CtlRef"=w507) -> ("FileUpToDate out"=w510:bool)  [unwired: 16 in]
            n372 = property on="FileUpToDate" class="Bool (strict)"("Value"=w510) -> ()  [unwired: 2 in, 2 out]
          }
          event "RetDisk1", "RetDisk2", "CoolWedge1", "CoolWedge2", "MicWedge1", "MicWedge2", "InjTunnel", "EndCool", "StartBun", "ExBun2", "DefLens", "BunDefX", "TranTube", "BunLens", "BunDefY", "Trap1Cool", "Trap1Eject", "Trap2Eject", "Trap2Cool", "Trap3Cool", "Trap3Eject", "Trap4Cool", "Trap4Eject", "Trap5Cool", "Trap5Eject", "Trap6Cool", "Trap7Cool", "Trap7Eject", "ExBun1Cool", "ExBun1Eject", "DCMicro", "DCBun", "DCCool", "Trap6Eject", "CoolPress", "AmpBun", "AmpMicro", "AmpCool": Value Change {
            # "Find sub-panel index"
            # "opening or closing a sub-panel"
            n373 = event-data() -> ("CtlRef"=w512:refnum<vi>)  [unwired: 1 in, 3 out]
            n374 = Search 1D Array(1D array=w513, element=w512) -> (index of element=w518:i32)  [unwired: 1 in]
            n375 = Index Array(array=w519, index=w518) -> (element=w516:refnum<vi>)
            n376 = invoke class="Bool" method="Reinit To Default"(reference=w512) -> ()  [unwired: 2 in, 3 out]
            n377 = property class="VI"(reference=w516) -> ("Front Panel.Open"=w515:bool)  [unwired: 1 in, 2 out]
            n378 = case "Panel Already Open?" shown="True" w515 {
              tunnel: w512 -> [w521 _]
              tunnel: w516 -> [_ w523]
              tunnel: [w520 refnum<vi> refnum ("vi reference")] -> w514
              frame False {
                n379 = call "OpenPanel.vi"("CtlRef"=w521) -> ("vi reference"=w520:refnum<vi>)  [unwired: 2 in]
              }
              frame True {
                n380 = call "PanelClose.vi"("vi reference"=w523) -> ()
              }
            }
            n381 = Replace Array Subset(array=w519, new element=w514, index=w518) -> (w517:refnum<vi>[])
          }
          event "Close All Panels": Value Change {
            n382 = event-data() -> ()  [unwired: 1 in, 6 out]
            n383 = case "Close Open Panels?" shown="True" "Close All Panels" {
              tunnel: w526 -> [w527 w529]
              tunnel: [w527 w528] -> w524
              frame False {
              }
              frame True {
                n384 = for "Close Open Panels" {
                  tunnel: w529 -> [w531] mode=indexing
                  tunnel: w529 -> [w530]
                  tunnel: [w530] -> w528
                  n385 = call "PanelClose.vi"("vi reference"=w531) -> ()
                }
              }
            }
          }
          event Timeout {
            # "Timeout"
            n386 = event-data() -> ()  [unwired: 1 in, 3 out]
          }
          event Panel Close? {
            n387 = event-data() -> ()  [unwired: 1 in, 4 out]
            n388 = stacked-sequence {
              tunnel: w536 -> [w542 _]
              tunnel: w535 -> [w541 _]
              tunnel: w534 -> [w540 _]
              tunnel: w533 -> [w544 _]
              frame #0 {
                # "Release DIM Services"
                n389 = for "Close Open Panels" {
                  tunnel: w544 -> [w554] mode=indexing
                  n390 = call "PanelClose.vi"("vi reference"=w554) -> ()
                }
                n391 = for "For Each Service" {
                  tunnel: w542 -> [w552] mode=indexing
                  n392 = Not A Number/Path/Refnum?(number/path/refnum=w552) -> (NaN/Path/Refnum?=w551:bool)
                  n393 = case "Not a Reference?" shown="False" w551 {
                    tunnel: w552 -> [w553 _]
                    frame False {
                      n394 = call "DimIndicators.dic_release_service.vi"("controlRef"=w553) -> ()  [unwired: 18 in, 1 out]
                    }
                    frame True {
                    }
                  }
                }
                n395 = for "For Each Service" {
                  tunnel: w541 -> [w549] mode=indexing
                  n396 = Not A Number/Path/Refnum?(number/path/refnum=w549) -> (NaN/Path/Refnum?=w548:bool)
                  n397 = case "Not a Reference?" shown="False" w548 {
                    tunnel: w549 -> [w550 _]
                    frame False {
                      n398 = call "DimIndicators.dic_release_service.vi"("controlRef"=w550) -> ()  [unwired: 18 in, 1 out]
                    }
                    frame True {
                    }
                  }
                }
                n399 = for "For Each Service" {
                  tunnel: w540 -> [w546] mode=indexing
                  n400 = Not A Number/Path/Refnum?(number/path/refnum=w546) -> (NaN/Path/Refnum?=w545:bool)
                  n401 = case "Not a Reference?" shown="False" w545 {
                    tunnel: w546 -> [w547 _]
                    frame False {
                      n402 = call "DimIndicators.dic_release_service.vi"("controlRef"=w547) -> ()  [unwired: 18 in, 1 out]
                    }
                    frame True {
                    }
                  }
                }
                n403 = control-ref of="ListOfBases_Data"() -> (w538:refnum<vi>)
                n404 = control-ref of="SetFileLocation_Data"() -> (w539:refnum<vi>)
                n405 = control-ref of="Last Loaded File_Data"() -> (w543:refnum<vi>)
                n406 = call "DimIndicators.dic_release_service.vi"("controlRef"=w538) -> ()  [unwired: 18 in, 1 out]
                n407 = call "DimIndicators.dic_release_service.vi"("controlRef"=w539) -> ()  [unwired: 18 in, 1 out]
                n408 = call "DimIndicators.dic_release_service.vi"("controlRef"=w543) -> ()  [unwired: 18 in, 1 out]
              }
              frame #1 {
                # "Close Front Panel"
                n409 = Current VI's Path() -> (path=w558:path)
                n410 = Open VI Reference(vi path=w558) -> (vi reference=w556:refnum<vi>, error out=w555:errorcluster)  [unwired: 5 in]
                n411 = property class="VI"(reference=w556, error in=w555, "Front Panel Window:Open"=FALSE) -> ()  [unwired: 2 out]
              }
            }
            n412 = event-data() -> ()  [unwired: 2 in, 1 out]
          }
        }
      }
    }
    frame #8 {
      n413 = stacked-sequence {
        tunnel: w562 -> [w565 _ _]
        tunnel: w561 -> [w569 _ _]
        tunnel: w560 -> [w566 _ _]
        tunnel: w559 -> [w567 _ _]
        frame #0 {
          # "Release DIM Services"
          n414 = control-ref of="Last Loaded File_Data"() -> (w568:refnum<vi>)
          n415 = control-ref of="SetFileLocation_Data"() -> (w564:refnum<vi>)
          n416 = control-ref of="ListOfBases_Data"() -> (w563:refnum<vi>)
          n417 = call "DimIndicators.dic_release_service.vi"("controlRef"=w563) -> ()  [unwired: 18 in, 1 out]
          n418 = call "DimIndicators.dic_release_service.vi"("controlRef"=w564) -> ()  [unwired: 18 in, 1 out]
          n419 = call "DimIndicators.dic_release_service.vi"("controlRef"=w568) -> ()  [unwired: 18 in, 1 out]
          n420 = for "For Each Service" {
            tunnel: w567 -> [w577] mode=indexing
            n421 = Not A Number/Path/Refnum?(number/path/refnum=w577) -> (NaN/Path/Refnum?=w576:bool)
            n422 = case "Not a Reference?" shown="False" w576 {
              tunnel: w577 -> [w578 _]
              frame False {
                n423 = call "DimIndicators.dic_release_service.vi"("controlRef"=w578) -> ()  [unwired: 18 in, 1 out]
              }
              frame True {
              }
            }
          }
          n424 = for "For Each Service" {
            tunnel: w566 -> [w574] mode=indexing
            n425 = Not A Number/Path/Refnum?(number/path/refnum=w574) -> (NaN/Path/Refnum?=w573:bool)
            n426 = case "Not a Reference?" shown="False" w573 {
              tunnel: w574 -> [w575 _]
              frame False {
                n427 = call "DimIndicators.dic_release_service.vi"("controlRef"=w575) -> ()  [unwired: 18 in, 1 out]
              }
              frame True {
              }
            }
          }
          n428 = for "For Each Service" {
            tunnel: [w570] -> _ mode=indexing
            tunnel: w565 -> [w570] mode=indexing
            n429 = Not A Number/Path/Refnum?(number/path/refnum=w570) -> (NaN/Path/Refnum?=w571:bool)
            n430 = case "Not a Reference?" shown="False" w571 {
              tunnel: w570 -> [w572 _]
              frame False {
                n431 = call "DimIndicators.dic_release_service.vi"("controlRef"=w572) -> ()  [unwired: 18 in, 1 out]
              }
              frame True {
              }
            }
          }
          n432 = for "Close Open Panels" {
            tunnel: w569 -> [w579] mode=indexing
            n433 = call "PanelClose.vi"("vi reference"=w579) -> ()
          }
        }
        frame #1 {
          # "Close Front Panel"
          n434 = Current VI's Path() -> (path=w583:path)
          n435 = Open VI Reference(vi path=w583) -> (vi reference=w581:refnum<vi>, error out=w580:errorcluster)  [unwired: 5 in]
          n436 = property class="VI"(reference=w581, error in=w580, "Front Panel Window:Open"=FALSE) -> ()  [unwired: 2 out]
        }
        frame #2 {
          # "Stop Panel"
          n437 = Stop(stop? (T)=TRUE) -> ()
        }
      }
    }
  }
  n438 = call "LVDimInterface.dim_operate.vi"("DNSNode"="lebit-balcony" ("DNS node")) -> ()  [unwired: 19 in]
